vi "ziExample-QControl.vi"() -> ()   [LabVIEW 2009]
doc: "Control a Zurich instrument device via the LabOne Labview API. \nRequirements: Zurich Instruments HF2LI with HF2-MF and HF2-PID options.\nThis LabVIEW vi helps in configuring an HF2 to do Q-Control.\n\n© Zurich Instruments AG, www.zhinst.com"
uses:
  <instrlib>/Zurich Instruments LabOne/Public/Configure/ziSetValueDouble.vi
  <vilib>/Analysis/NI_AALPro.lvlib
  <vilib>/Utility/NIReport.llb/NI_report.lvclass
  <instrlib>/Zurich Instruments LabOne/Zurich Instruments LabOne.lvlib
panel:
  in  "restore settings":bool caption="Restore original settings"
  out "fmax":dbl=1000.0
  out "fmin":dbl=1000.0
  in  "Tab Control Sweep":enum32{"Sweeper", "Sweeper Settings", "Help"}(tab)
  in  "Drive (V)":dbl=0.01 format="%_3p"
  out "Resonance Frequency Q":dbl
  in  "Run Sweep":bool
  out "Sweep Progress":dbl(slide) max=21.0 scale=0.0..1.0
  out "Graph Phase":T1(graph)=[{"Output (F,X1,Y1,X2,Y2,...,Vo)"=[1841839.1959798995, 1841849.2462311557, 1841859.2964824121, 1841869.3467336684, 1841879.3969849246, 1841889.447236181, 1841899.4974874372, 1841909.5477386934, 1841919.5979899496, 1841929.648241206, 1841939.6984924623, 1841949.7487437185, 1841959.798994975, 1841969.8492462311, 1841979.8994974873, 1841989.9497487438, 1842000.0, 1842010.0502512562, 1842020.1005025127, 1842030.1507537689, 1842040.201005025, 1842050.2512562815, 1842060.3015075377, 1842070.351758794, 1842080.4020100501, 1842090.4522613066, 1842100.5025125628, 1842110.552763819, 1842120.6030150754, 1842130.6532663316, 1842140.7035175879, 1842150.7537688443, 1842160.8040201005, 1842170.8542713567, 1842180.9045226132, 1842190.9547738694, 1842201.0050251256, 1842211.055276382, 1842221.1055276382, 1842231.1557788944, 1842241.2060301506, 1842251.256281407, 1842261.3065326633, 1842271.3567839195, 1842281.407035176, 1842291.4572864322, 1842301.5075376884, 1842311.5577889448, 1842321.608040201, 1842331.6582914572, 1842341.7085427137, 1842351.7587939699, 1842361.809045226, 1842371.8592964825, 1842381.9095477387, 1842391.959798995, 1842402.0100502511, 1842412.0603015076, 1842422.1105527638, 1842432.16080402, 1842442.2110552764, 1842452.2613065327, 1842462.3115577889, 1842472.3618090453, 1842482.4120603015, 1842492.4623115577, 1842502.5125628142, 1842512.5628140704, 1842522.6130653266, 1842532.6633165828, 1842542.7135678392, 1842552.7638190954, 1842562.8140703517, 1842572.864321608, 1842582.9145728643, 1842592.9648241205, 1842603.015075377, 1842613.0653266332, 1842623.1155778894, 1842633.1658291458, 1842643.216080402, 1842653.2663316582, 1842663.3165829147, 1842673.3668341709, 1842683.417085427, 1842693.4673366833, 1842703.5175879397, 1842713.567839196, 1842723.6180904522, 1842733.6683417086, 1842743.7185929648, 1842753.768844221, 1842763.8190954775, 1842773.8693467337, 1842783.9195979899, 1842793.9698492463, 1842804.0201005025, 1842814.0703517587, 1842824.1206030152, 1842834.1708542714, 1842844.2211055276, 1842854.2713567838, 1842864.3216080402, 1842874.3718592965, 1842884.4221105527, 1842894.472361809, 1842904.5226130653, 1842914.5728643215, 1842924.623115578, 1842934.6733668342, 1842944.7236180904, 1842954.7738693468, 1842964.824120603, 1842974.8743718592, 1842984.9246231157, 1842994.974874372, 1843005.025125628, 1843015.0753768843, 1843025.1256281408, 1843035.175879397, 1843045.2261306532, 1843055.2763819096, 1843065.3266331658, 1843075.376884422, 1843085.4271356785, 1843095.4773869347, 1843105.527638191, 1843115.5778894473, 1843125.6281407035, 1843135.6783919598, 1843145.7286432162, 1843155.7788944724, 1843165.8291457286, 1843175.8793969848, 1843185.9296482413, 1843195.9798994975, 1843206.0301507537, 1843216.0804020101, 1843226.1306532663, 1843236.1809045225, 1843246.231155779, 1843256.2814070352, 1843266.3316582914, 1843276.3819095478, 1843286.432160804, 1843296.4824120603, 1843306.5326633165, 1843316.582914573, 1843326.6331658291, 1843336.6834170853, 1843346.7336683418, 1843356.783919598, 1843366.8341708542, 1843376.8844221106, 1843386.9346733668, 1843396.984924623, 1843407.0351758795, 1843417.0854271357, 1843427.135678392, 1843437.1859296483, 1843447.2361809046, 1843457.2864321608, 1843467.336683417, 1843477.3869346734, 1843487.4371859296, 1843497.4874371858, 1843507.5376884423, 1843517.5879396985, 1843527.6381909547, 1843537.6884422111, 1843547.7386934673, 1843557.7889447236, 1843567.83919598, 1843577.8894472362, 1843587.9396984924, 1843597.9899497489, 1843608.040201005, 1843618.0904522613, 1843628.1407035175, 1843638.190954774, 1843648.2412060301, 1843658.2914572863, 1843668.3417085428, 1843678.391959799, 1843688.4422110552, 1843698.4924623116, 1843708.5427135678, 1843718.592964824, 1843728.6432160805, 1843738.6934673367, 1843748.743718593, 1843758.7939698494, 1843768.8442211056, 1843778.8944723618, 1843788.944723618, 1843798.9949748744, 1843809.0452261306, 1843819.0954773868, 1843829.1457286433, 1843839.1959798995], "dX/dt"=[-6.94293659208085, -7.039263365714603, -7.015747865746605, -7.022831577183382, -7.070140649231355, -7.097687461922305, -7.105617775743133, -7.187018771027357, -7.215555605807255, -7.209120372797453, -7.222963353111247, -7.2482145424437725, -7.336471988299522, -7.392871009974112, -7.404378015656745, -7.392520359287413, -7.520355608686046, -7.519542598388936, -7.550628880706965, -7.581504623203495, -7.613602056591421, -7.5885724211422065, -7.700014320037284, -7.728140979121345, -7.810709171761543, -7.784263466588973, -7.881518062030821, -7.903674328964446, -7.971719351332499, -8.017529667992314, -8.058121436672986, -8.165785698106287, -8.19016022550502, -8.212700433959935, -8.32675261509468, -8.371215456694097, -8.455244319826404, -8.452589972505562, -8.593897328803308, -8.603598584374405, -8.66788383890823, -8.728838589412112, -8.92008246055265, -8.96248928060953, -9.014325061381626, -9.12099819745259, -9.192260387685824, -9.25577287991073, -9.393754573052911, -9.510460418962696, -9.588798588744128, -9.671919305255168, -9.807909390069907, -9.872318951901494, -10.029523543826793, -10.111178612582068, -10.282365199143047, -10.41392827403316, -10.600908552099941, -10.721664299953895, -10.861537419641733, -11.05386683133099, -11.226967260541015, -11.399833261360014, -11.614266576451872, -11.822489241822097, -12.037591738878548, -12.284275795570396, -12.537696676929697, -12.808591866080967, -13.10897592112657, -13.414554360121997, -13.74678013981217, -14.102456694459267, -14.476936500710565, -14.894674114827959, -15.339877668460199, -15.812096714688613, -16.374409982820275, -16.9513079644051, -17.5854888581396, -18.28427561683263, -19.054069906143813, -19.928879874410452, -20.90995289279427, -21.975478569369823, -23.22079284159497, -24.61324931082536, -26.23607602255107, -28.12290317293296, -30.316540859101774, -32.93351414204068, -36.0685114581311, -39.86225308894581, -44.52062048412513, -50.265070638918324, -57.397192144852305, -66.16528396414377, -76.63221848917898, -88.4706687072364, -100.82403856696656, -112.6132379050097, -122.9993546962758, -131.68277440223207, -138.73027439508525, -144.42272136521782, -149.00962859772702, -152.74574201067415, -155.83478009073983, -158.4057569715815, -160.55712878950192, -162.41389955531858, -163.98916270213934, -165.35435338829546, -166.5502332885727, -167.6188034018421, -168.54149862098475, -169.38780172777604, -170.13679818450444, -170.78748418559624, -171.41172295788104, -171.99098890699028, -172.50066268325997, -172.9556325234782, -173.4008952713357, -173.82760697801268, -174.17343776744914, -174.55598606411053, -174.82677313412782, -175.20114654856826, -175.44438260372488, -175.74183048219098, -176.00347473058068, -176.23123546164112, -176.43388652935894, -176.62506543519825, -176.8656495868036, -177.000286426292, -177.2712077683475, -177.36028159834026, -177.53319063513797, -177.67555828450963, -177.84294696805748, -178.0118748631806, -178.16232009535963, -178.27551219372313, -178.39423075255817, -178.4903282214428, -178.5715733424731, -178.73836280736876, -178.82943056728186, -178.9850843467714, -179.04192894715334, -179.08270482893664, -179.19287748311572, -179.28322843883868, -179.34165759880761, -179.50709018669053, -179.4954309299658, -179.64736857972363, -179.60928252514617, -179.78420449956272, -179.8065606796536, -179.84218357544378, -179.90164268987297, -179.9062773498495, -180.0402030141334, -180.21011520251875, -180.02003421747088, -180.17501517626974, -180.197905755971, -180.35296807746022, -180.37609298337136, -180.54331181359302, -180.49811587577673, -180.50365280444166, -180.6359768081795, -180.47976323601006, -180.5713600449198, -180.67329316815656, -180.6154046528325, -180.75094639042254, -180.5940820677559, -180.83667931766678, -180.72000977161738, -180.90668274161465, -180.88415063790313, -180.91032933351386, -180.93791455694205, -180.8862600292335, -180.9706632041318, -181.0058055371726, -181.12385131631882, -180.99226180353708, -181.17117500602515, -181.20440954183448, -181.1560016539221, -181.11269108982725, -181.29568987605847, -181.260867961045]}, {"Output (F,X1,Y1,X2,Y2,...,Vo)"=array[500 elements], "dX/dt"=array[500 elements]}] caption="Graph2"
  out "Graph Amplitude":T2(graph)=[{"Output (F,X1,Y1,X2,Y2,...,Vo)"=[1841839.1959798995, 1841849.2462311557, 1841859.2964824121, 1841869.3467336684, 1841879.3969849246, 1841889.447236181, 1841899.4974874372, 1841909.5477386934, 1841919.5979899496, 1841929.648241206, 1841939.6984924623, 1841949.7487437185, 1841959.798994975, 1841969.8492462311, 1841979.8994974873, 1841989.9497487438, 1842000.0, 1842010.0502512562, 1842020.1005025127, 1842030.1507537689, 1842040.201005025, 1842050.2512562815, 1842060.3015075377, 1842070.351758794, 1842080.4020100501, 1842090.4522613066, 1842100.5025125628, 1842110.552763819, 1842120.6030150754, 1842130.6532663316, 1842140.7035175879, 1842150.7537688443, 1842160.8040201005, 1842170.8542713567, 1842180.9045226132, 1842190.9547738694, 1842201.0050251256, 1842211.055276382, 1842221.1055276382, 1842231.1557788944, 1842241.2060301506, 1842251.256281407, 1842261.3065326633, 1842271.3567839195, 1842281.407035176, 1842291.4572864322, 1842301.5075376884, 1842311.5577889448, 1842321.608040201, 1842331.6582914572, 1842341.7085427137, 1842351.7587939699, 1842361.809045226, 1842371.8592964825, 1842381.9095477387, 1842391.959798995, 1842402.0100502511, 1842412.0603015076, 1842422.1105527638, 1842432.16080402, 1842442.2110552764, 1842452.2613065327, 1842462.3115577889, 1842472.3618090453, 1842482.4120603015, 1842492.4623115577, 1842502.5125628142, 1842512.5628140704, 1842522.6130653266, 1842532.6633165828, 1842542.7135678392, 1842552.7638190954, 1842562.8140703517, 1842572.864321608, 1842582.9145728643, 1842592.9648241205, 1842603.015075377, 1842613.0653266332, 1842623.1155778894, 1842633.1658291458, 1842643.216080402, 1842653.2663316582, 1842663.3165829147, 1842673.3668341709, 1842683.417085427, 1842693.4673366833, 1842703.5175879397, 1842713.567839196, 1842723.6180904522, 1842733.6683417086, 1842743.7185929648, 1842753.768844221, 1842763.8190954775, 1842773.8693467337, 1842783.9195979899, 1842793.9698492463, 1842804.0201005025, 1842814.0703517587, 1842824.1206030152, 1842834.1708542714, 1842844.2211055276, 1842854.2713567838, 1842864.3216080402, 1842874.3718592965, 1842884.4221105527, 1842894.472361809, 1842904.5226130653, 1842914.5728643215, 1842924.623115578, 1842934.6733668342, 1842944.7236180904, 1842954.7738693468, 1842964.824120603, 1842974.8743718592, 1842984.9246231157, 1842994.974874372, 1843005.025125628, 1843015.0753768843, 1843025.1256281408, 1843035.175879397, 1843045.2261306532, 1843055.2763819096, 1843065.3266331658, 1843075.376884422, 1843085.4271356785, 1843095.4773869347, 1843105.527638191, 1843115.5778894473, 1843125.6281407035, 1843135.6783919598, 1843145.7286432162, 1843155.7788944724, 1843165.8291457286, 1843175.8793969848, 1843185.9296482413, 1843195.9798994975, 1843206.0301507537, 1843216.0804020101, 1843226.1306532663, 1843236.1809045225, 1843246.231155779, 1843256.2814070352, 1843266.3316582914, 1843276.3819095478, 1843286.432160804, 1843296.4824120603, 1843306.5326633165, 1843316.582914573, 1843326.6331658291, 1843336.6834170853, 1843346.7336683418, 1843356.783919598, 1843366.8341708542, 1843376.8844221106, 1843386.9346733668, 1843396.984924623, 1843407.0351758795, 1843417.0854271357, 1843427.135678392, 1843437.1859296483, 1843447.2361809046, 1843457.2864321608, 1843467.336683417, 1843477.3869346734, 1843487.4371859296, 1843497.4874371858, 1843507.5376884423, 1843517.5879396985, 1843527.6381909547, 1843537.6884422111, 1843547.7386934673, 1843557.7889447236, 1843567.83919598, 1843577.8894472362, 1843587.9396984924, 1843597.9899497489, 1843608.040201005, 1843618.0904522613, 1843628.1407035175, 1843638.190954774, 1843648.2412060301, 1843658.2914572863, 1843668.3417085428, 1843678.391959799, 1843688.4422110552, 1843698.4924623116, 1843708.5427135678, 1843718.592964824, 1843728.6432160805, 1843738.6934673367, 1843748.743718593, 1843758.7939698494, 1843768.8442211056, 1843778.8944723618, 1843788.944723618, 1843798.9949748744, 1843809.0452261306, 1843819.0954773868, 1843829.1457286433, 1843839.1959798995], [-28.966250862681054, -28.908176655273337, -28.864467111398284, -28.808136126619875, -28.754602779877295, -28.681537195962324, -28.60547886691201, -28.542769551012277, -28.47986278834069, -28.413059310021236, -28.35033543586046, -28.29138537216195, -28.227086468764178, -28.15168084424244, -28.083132309459675, -28.006652538062877, -27.923391524657678, -27.862916544212467, -27.784208516740375, -27.70412391696607, -27.636354468592554, -27.55133643843743, -27.46146332129707, -27.389341692048106, -27.294868081757663, -27.219310281261595, -27.123230188479226, -27.03474855024407, -26.950586594813416, -26.85355121081612, -26.765683710166535, -26.675242143760556, -26.564063048008382, -26.474632733618588, -26.37565770196402, -26.280112494285053, -26.172991235949205, -26.072598624000236, -25.959534728054443, -25.860640493819343, -25.7465174301761, -25.631539306182212, -25.498858352667277, -25.39010824649092, -25.25774799718558, -25.142249321882026, -25.00555406360646, -24.887022970441244, -24.75211169976204, -24.617521743246748, -24.48274082231197, -24.3428232828688, -24.196009592241655, -24.047554642475653, -23.889297411413008, -23.739575356461376, -23.570294117173674, -23.41322125110465, -23.224954797726845, -23.058866498583328, -22.88382952274905, -22.69856576681898, -22.50867999213655, -22.31450162319383, -22.111370069423263, -21.90338344600061, -21.68504571797671, -21.461764169109074, -21.226543135169543, -20.99229287484784, -20.741801499413626, -20.479366183700762, -20.21176825406491, -19.937742640458776, -19.648956986305464, -19.3468251889951, -19.033496520395904, -18.701812675964042, -18.355682042916765, -17.99270040419432, -17.615604660651464, -17.21865908953786, -16.797539016940565, -16.356977304926286, -15.888200014085553, -15.391846986851675, -14.866834628179921, -14.309077261379437, -13.711689066706123, -13.074653632558586, -12.392712546398329, -11.663574717432795, -10.884371326060215, -10.054211061904741, -9.183959621011658, -8.284378130216394, -7.3946969716815065, -6.579866401883259, -5.946660172340811, -5.612275426625389, -5.660939792976745, -6.092597885403304, -6.819063594921346, -7.720596881253953, -8.692845639671399, -9.676601274917646, -10.63194093311314, -11.542743236475578, -12.406298891129273, -13.216035317601213, -13.98028024462563, -14.699677218013587, -15.379521411615144, -16.023339805333272, -16.632012788033276, -17.212135663274463, -17.763951487592156, -18.287404341430125, -18.79046016208909, -19.273915407845625, -19.736440474832023, -20.179725827914766, -20.608959575656495, -21.018134587427294, -21.422995318238737, -21.807627924716133, -22.17859768043806, -22.532821774822636, -22.88528270717979, -23.228299264102954, -23.55688511871147, -23.881717376684854, -24.19613894993444, -24.49895105674716, -24.802029226261308, -25.099837529936202, -25.392446478391577, -25.673862567600672, -25.947515476929528, -26.22420324643256, -26.473552872567087, -26.742550094460967, -27.00104527827544, -27.248345780939687, -27.491641603363373, -27.74480782051559, -27.98078562862448, -28.223226877341677, -28.4458543248418, -28.668372965623256, -28.91316733771661, -29.134686427564475, -29.34772484111448, -29.55621510607997, -29.784051895982245, -30.00136613401197, -30.219876575206612, -30.42218292074636, -30.618607334447535, -30.831568097485093, -31.031377814888664, -31.230073398030804, -31.42672173766795, -31.62404980158688, -31.819935098980814, -32.01368910890594, -32.20561075361435, -32.396695113595065, -32.58604024745495, -32.754436974363834, -32.96100063832588, -33.124166975360936, -33.323942883117475, -33.50090098141094, -33.683801355462585, -33.87460045378752, -34.03049976000201, -34.25189149349637, -34.40356326157614, -34.580744989166725, -34.75748170316221, -34.94748867729741, -35.11731073350964, -35.288783018518025, -35.44821022332193, -35.6213094778834, -35.8056140321162, -35.95929649243196, -36.124591783023774, -36.30593369611333, -36.503240497902596, -36.64816967067446, -36.79128348867193, -36.99164183710858, -37.143384953777364, -37.26823219562254, -37.49034966949507, -37.662154614518144, -37.81959794162762, -38.00695446481112]}, {"Output (F,X1,Y1,X2,Y2,...,Vo)"=array[500 elements], array[500 elements]}] caption="Graph1"
  out "Q Factor":dbl format="%_4f"
  out "Resonance Freq (Hz)":dbl
  out "Phase Shift (°)":dbl format="%#.2f"
  out "controlled":dbl format="%_4f"
  out "Gain Margin (dB)":dbl caption="native" format="%.2f"
  out "f/2Q (Hz)":dbl
  out "Characteristic Frequency Q":dbl
  in  "Output Demod":i32(ring)=6 items=["1", "2", "3", "4", "5", "6", "7", "8"]
  in  "Steps":dbl=100.0
  in  "BW (Hz)":dbl=500.0
  in  "AutoBW":bool caption="Auto"
  in  "Sweep Oscillator":i32(ring) caption="Oscillator" items=["1", "2", "3", "4", "5", "6"]
  in  "Show Derivative and Filter":bool caption="Show demodulator filter and phase derivative in graphs"
  in  "Tab Control QControl":T3(tab)
  in  "PID Drive Limit (V)":dbl=10.0 format="%.3g"
  in  "Center Frequency (Hz)":dbl=1000000.0 format="%#_8p"
  in  "Bandwidth (Hz)":dbl=1000.0 format="%#_4p"
  in  "Q Control En":bool caption="Enable"
  in  "HW Channel":i32(ring) caption="Signal Input and Output" items=["1", "2"]
  in  "Q Enhancement":dbl(slide) scale=0.1..100.0 scale format="%#_4g"
  in  "AutoCenter":bool caption="Auto Center"
  in  "Address":string="DEV"
  out "Selected Device":string
  in  "PIDs":i32(ring) items=["1 and 2", "3 and 4"]
  in  "Oscillator":i32(ring)=2 items=["1", "2", "3", "4", "5", "6"]
  in  "Feedback Phase (deg)":dbl(slide) scale=-180.0..180.0
  in  "Feedback Gain (V/Vrms)":dbl(slide) scale=0.01..100.0
  out "Stability Warning":bool
  in  "AutoPhase":bool caption="Auto"
  in  "Auto Gain":bool caption="Auto"
  out "ADC Over":bool
  in  "stop":bool
  # "Requires HF2LI or MFLI with MF and PID options."
  # "Beta user help:\n1) Connect the resonator to either Signal Output 1 and Signal Input 1 or to both #2.\n\n2) Find out the approximate resonator resonance frequency and enter it to the field \"Center Frequency\"\n\n3) Specify \"Bandwidth\" to be about 5x the width of the resonance peak (*).\n\n4) Start a sweep to find the native (natural) behavior of the resonator. The exact resonance frequency, Q-factor, characteristic frequency, phase at resonance and gain margin will be extracted. These values are crucial for a proper Q enhancement. (**)\n\n5) Set the \"Q Enhancement\" slider to the desired value (2 increases Q by a factor of two) and enable Q control.\n\n6) Start another sweep and compare the transfer functions.\n\n* Keep in mind that the resonance may not shift more than the Q-control bandwidth. Bandwidth should not be set to a higher value than 10kHz as the PID controllers can update the drive with about 100kHz.\n** The time constant setting for the sweeper should suit the characteristic frequency of the cantilever."
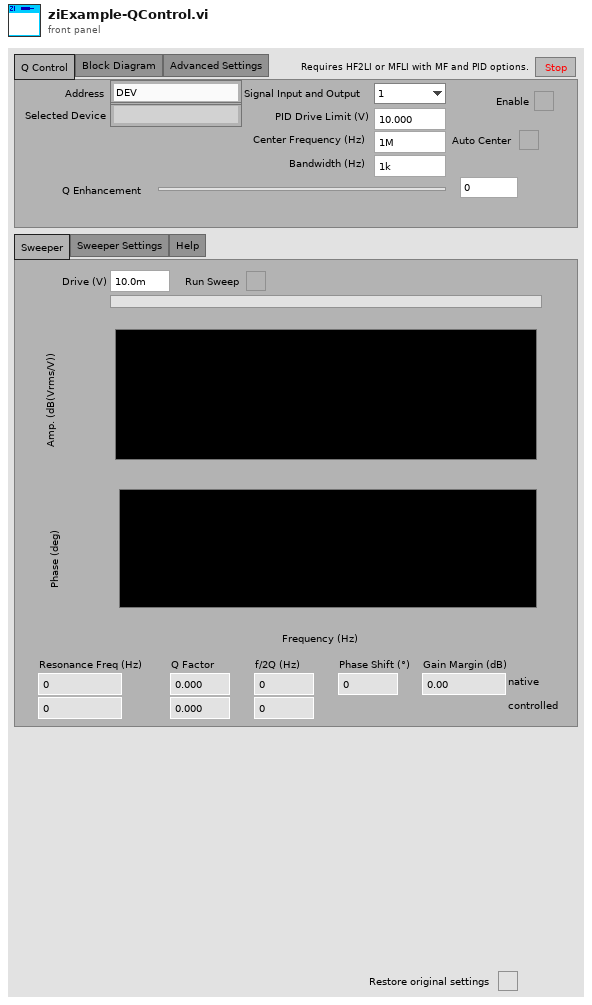
[diagram p1: front panel]
types:
  T1 = cluster{"Output (F,X1,Y1,X2,Y2,...,Vo)":dbl[], "dX/dt":dbl[]}[]
  T2 = cluster{"Output (F,X1,Y1,X2,Y2,...,Vo)":dbl[], dbl[]}[]
  T3 = enum32{"Q Control", "Block Diagram", "Advanced Settings"}
  T4 = enum32{"Page Enabled", "Page Disabled", "Page Disabled & Grayed"}
  T5 = enum8{"Enabled", "Disabled", "Disabled and Grayed Out"}
  T6 = typedef "Zurich Instruments LabOne.lvlib/ziTypeHandle.ctl" = cluster{"handleValid":bool, "Conn":u64, "Path Prefix":string, "Handle":u64, "Connected":bool, "Clockbase(s)":dbl}
  T7 = enum16{"Standard Report", "HTML", "Word", "Excel"}
  T8 = cluster{"Output (F,X1,Y1,X2,Y2,...,Vo)":dbl[], dbl[]}
  T9 = cluster{"Output (F,X1,Y1,X2,Y2,...,Vo)":dbl[], "Unwrapped Phase":dbl[]}
  T10 = enum32{"invalid app kind", "Development System", "Run Time System", "Student Edition", "Embedded LabVIEW", "Evaluation", "Custom"}
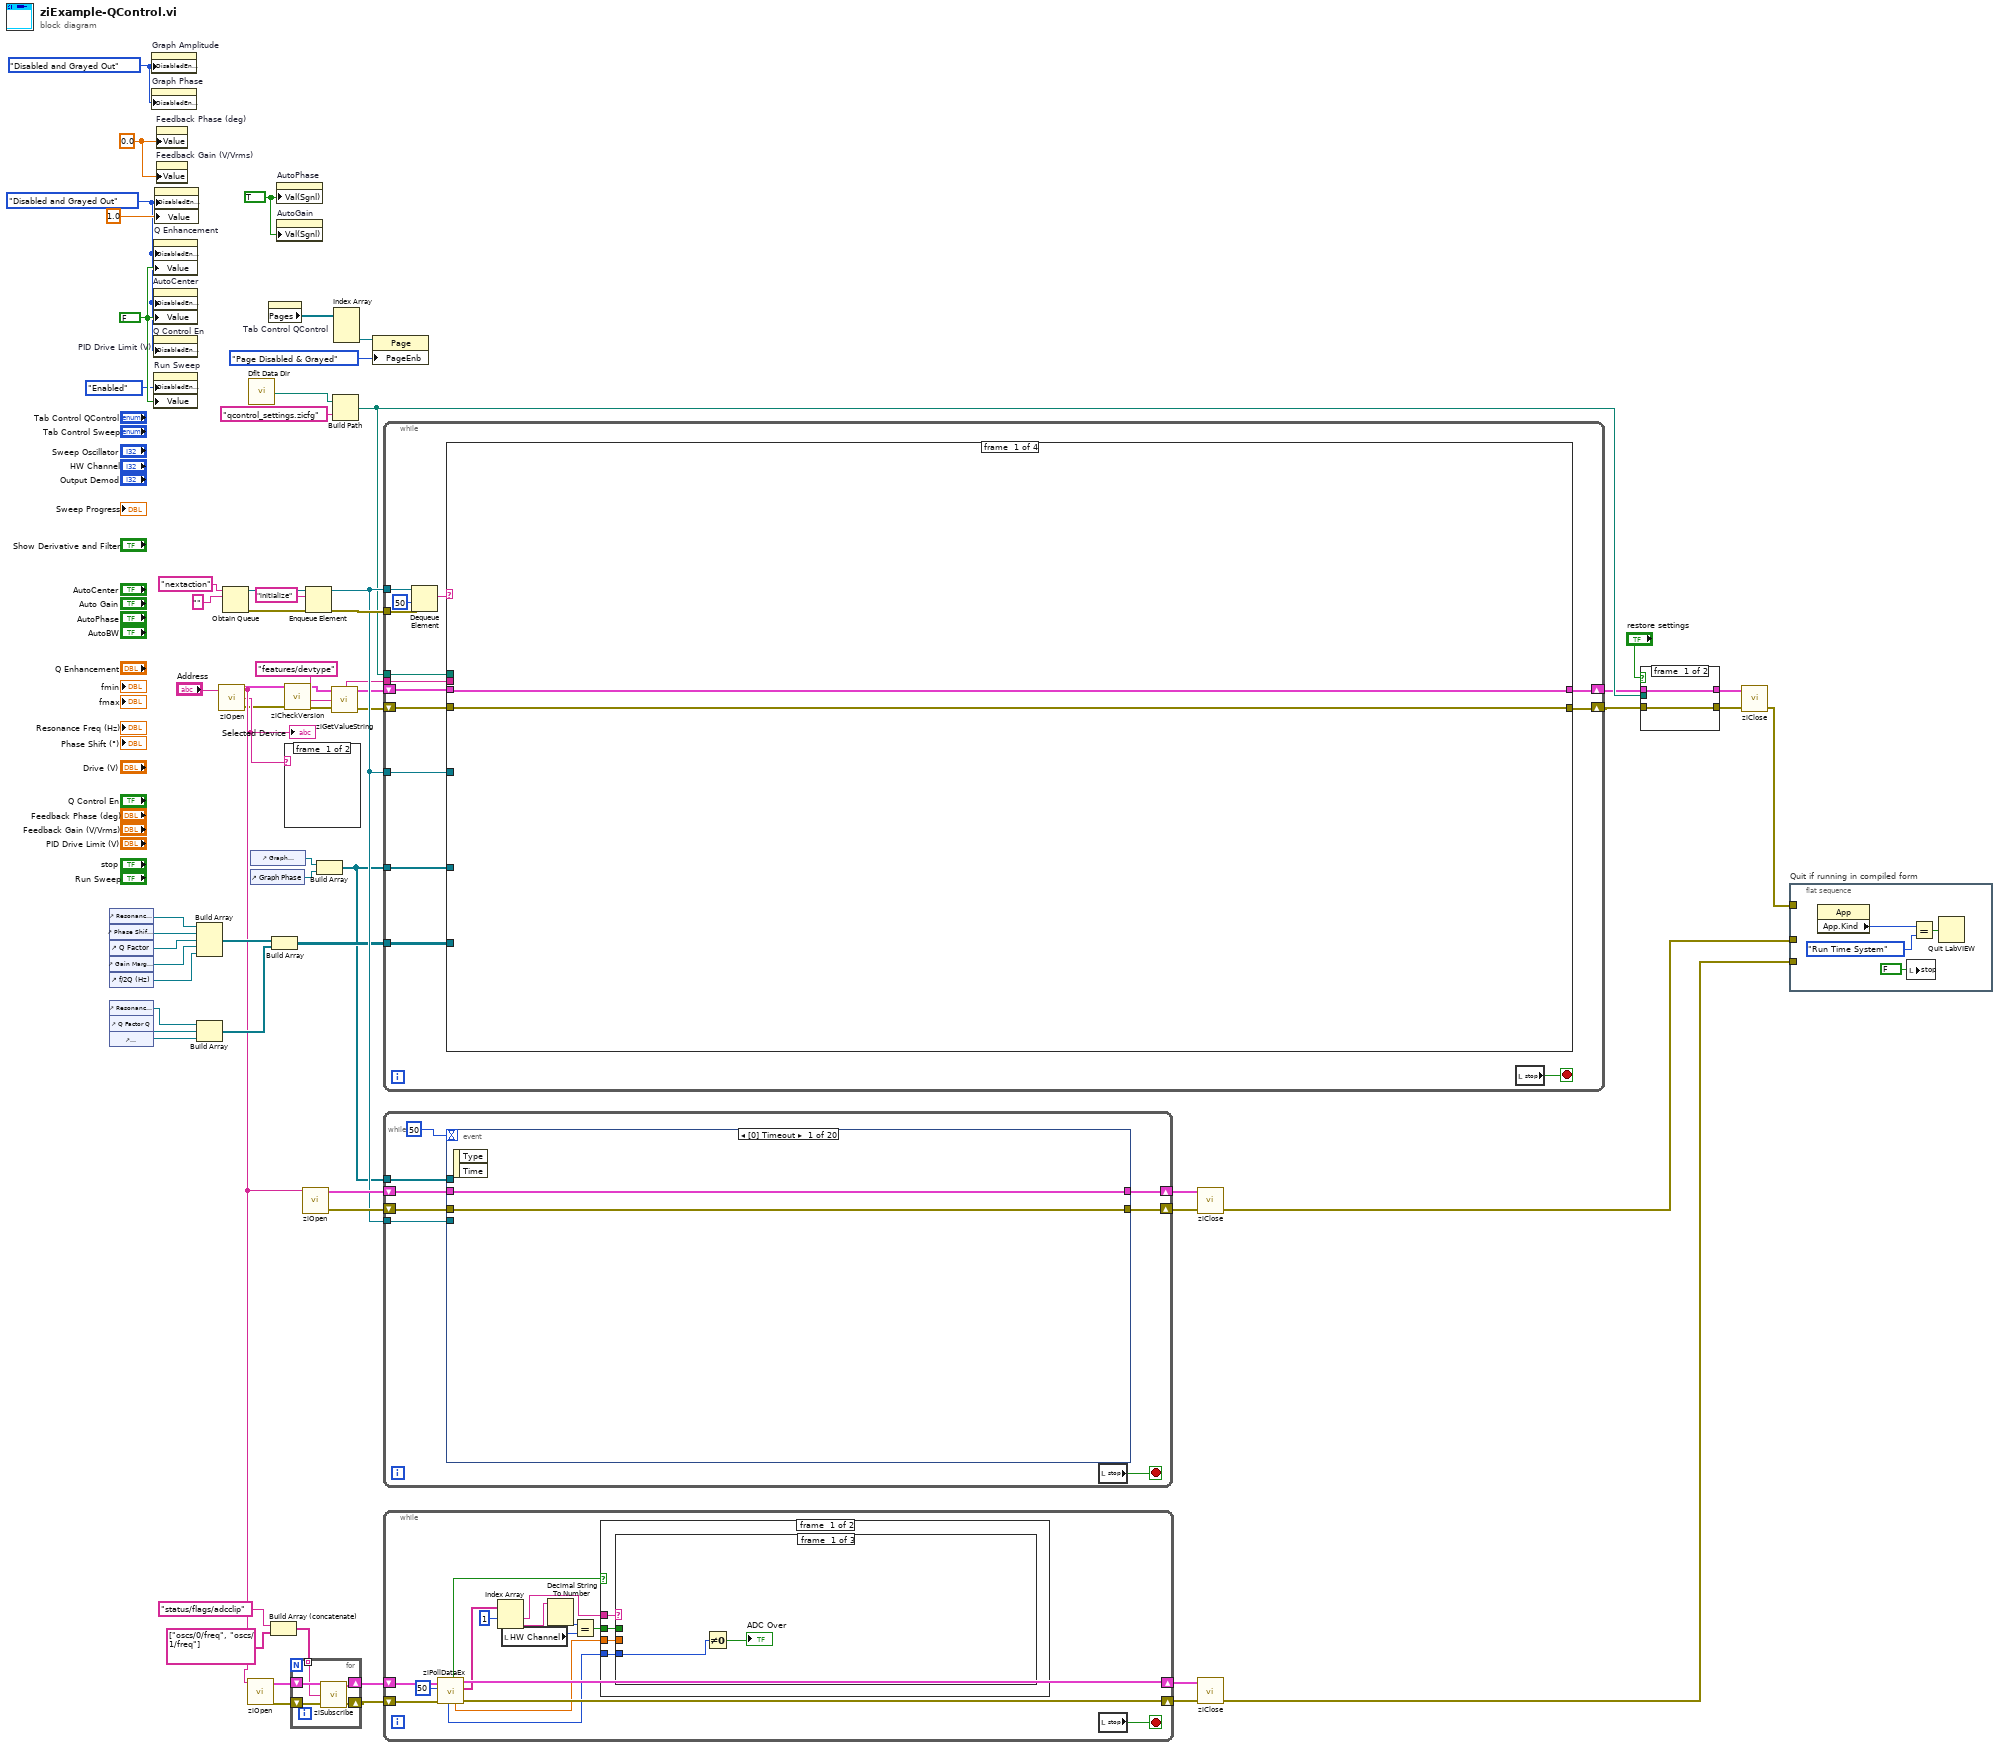
[diagram p0: block diagram]
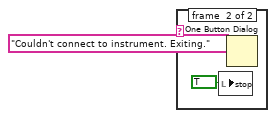
[diagram p2: hidden frame]
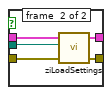
[diagram p3: hidden frame]
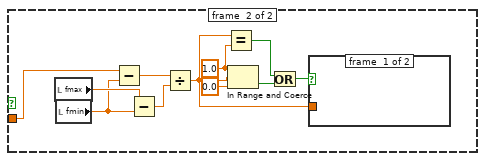
[diagram p6: hidden frame]
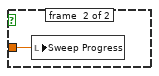
[diagram p7: hidden frame]
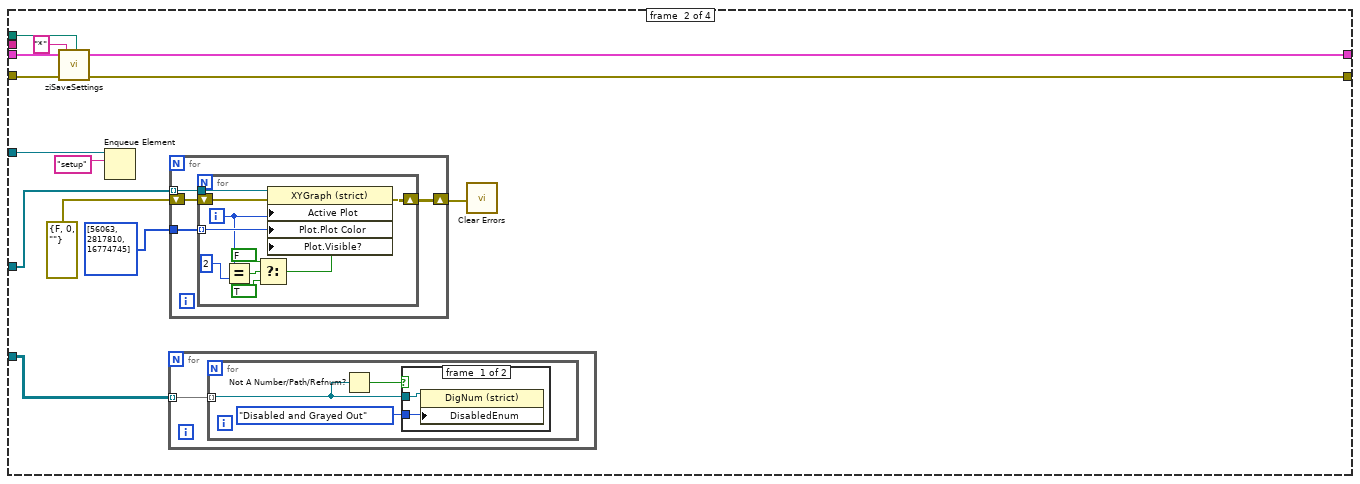
[diagram p9: hidden frame]
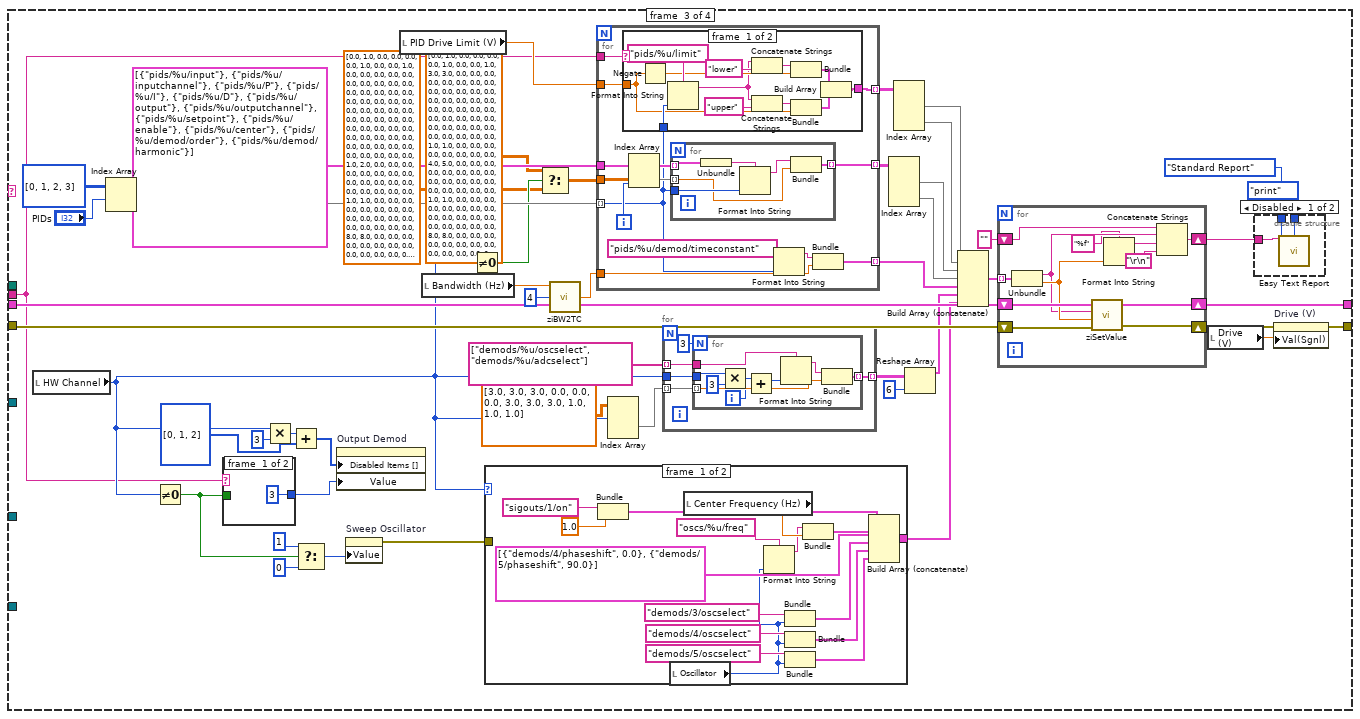
[diagram p11: hidden frame]
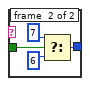
[diagram p12: hidden frame]
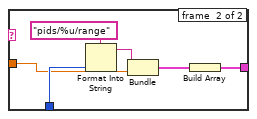
[diagram p14: hidden frame]
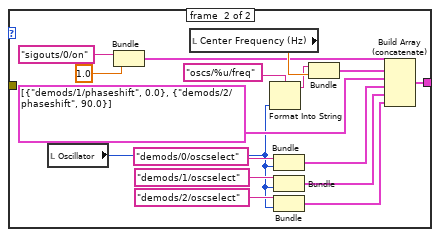
[diagram p15: hidden frame]
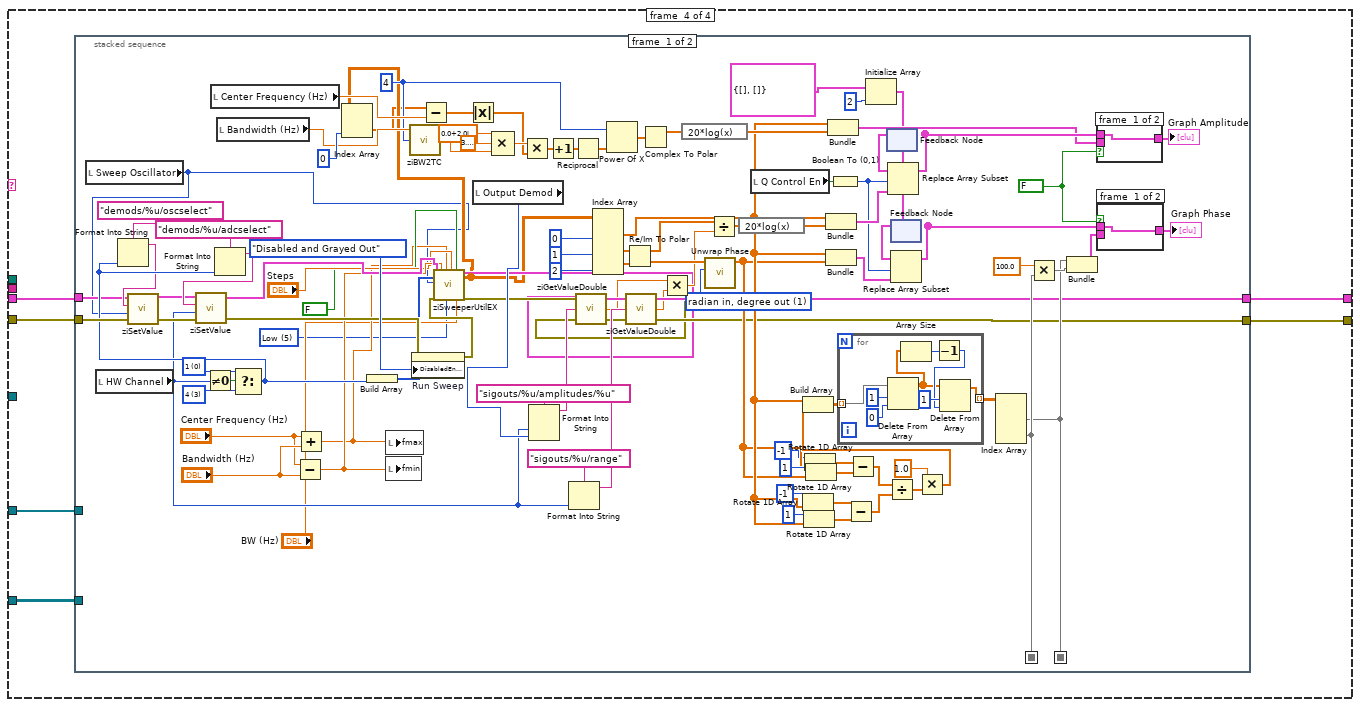
[diagram p16: hidden frame]
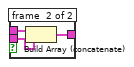
[diagram p17: hidden frame]
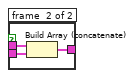
[diagram p18: hidden frame]
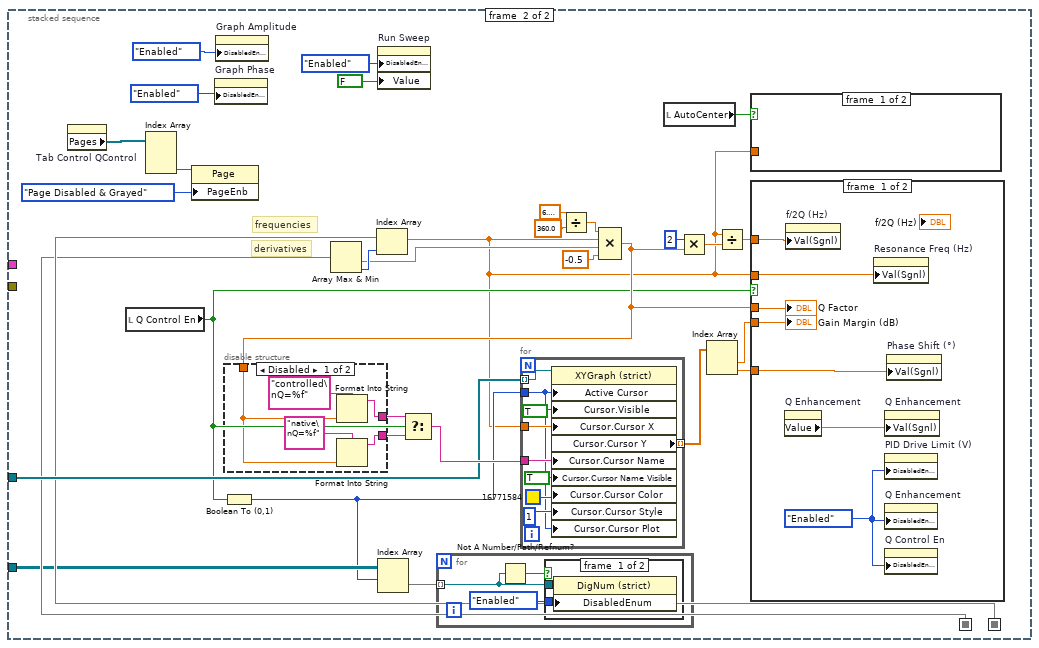
[diagram p19: hidden frame]
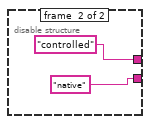
[diagram p20: hidden frame]
diagram:
  w6 = T5."Disabled and Grayed Out" ("Disabled")
  w17 = 0.0 ("Feedback Phase (deg)")
  w18 = TRUE ("AutoPhase")
  w5 = T5."Disabled and Grayed Out" ("Disabled")
  w20 = FALSE ("Q Control")
  n1 = control-ref of="Resonance Freq (Hz)"() -> (w50:refnum<vi>)
  n2 = control-ref of="Phase Shift (°)"() -> (w49:refnum<vi>)
  n3 = control-ref of="Q Factor"() -> (w48:refnum<vi>)
  n4 = control-ref of="Gain Margin (dB)"() -> (w47:refnum<vi>)
  n5 = control-ref of="f/2Q (Hz)"() -> (w40:refnum<vi>)
  n6 = control-ref of="Resonance Frequency Q"() -> (w38:refnum<vi>)
  n7 = control-ref of="Q Factor Q"() -> (w46:refnum<vi>)
  n8 = control-ref of="Characteristic Frequency Q"() -> (w39:refnum<vi>)
  n9 = property on="Graph Amplitude" class="XYGraph (strict)"("DisabledEnum"=w6) -> ()  [unwired: 2 in, 2 out]
  n10 = property on="Graph Phase" class="XYGraph (strict)"("DisabledEnum"=w6) -> ()  [unwired: 2 in, 2 out]
  n11 = property on="AutoCenter" class="Bool (strict)"("DisabledEnum"=w5, "Value"=w20) -> ()  [unwired: 2 in, 2 out]
  n12 = property on="Q Control En" class="Bool (strict)"("DisabledEnum"=w5, "Value"=w20) -> ()  [unwired: 2 in, 2 out]
  n13 = property on="PID Drive Limit (V)" class="DigNum (strict)"("DisabledEnum"=w5) -> ()  [unwired: 2 in, 2 out]
  n14 = property on="Run Sweep" class="Bool (strict)"("DisabledEnum"=T5."Enabled" ("Disabled"), "Value"=w20) -> ()  [unwired: 2 in, 2 out]
  n15 = property on="Q Enhancement" class="Slide (strict)"("DisabledEnum"=w5, "Value"=1.0 ("Q Enhancement")) -> ()  [unwired: 2 in, 2 out]
  n16 = property on="Feedback Phase (deg)" class="Slide (strict)"("Value"=w17) -> ()  [unwired: 2 in, 2 out]
  n17 = property on="Feedback Gain (V/Vrms)" class="Slide (strict)"("Value"=w17) -> ()  [unwired: 2 in, 2 out]
  n18 = Build Array(w50, w49, w48, w47, w40) -> (w44:refnum<vi>[])
  n19 = Build Array(w38, w46, w39) -> (w45:refnum<vi>[])
  n20 = call <instrlib>:"ziOpen.vi"("Address"="Address") -> ("Error Out"=w1:errorcluster, "Selected Device"=w8:string, "HandleOut"=w2:T6)  [unwired: 3 in]
  "Selected Device" <- w8
  n21 = Obtain Queue(name (unnamed)="nextaction", element data type="") -> (queue out=w63:refnum<queue>, error out=w61:errorcluster)  [unwired: 3 in, 1 out]
  n22 = call <instrlib>:"ziOpen.vi"("Address"="Address") -> ("Error Out"=w51:errorcluster, "HandleOut"=w52:T6)  [unwired: 3 in, 1 out]
  n23 = call <vilib>:"Dflt Data Dir.vi"() -> ("App:Default Data Directory"=w37:path)
  n24 = control-ref of="Graph Phase"() -> (w41:refnum<vi>)
  n25 = control-ref of="Graph Amplitude"() -> (w42:refnum<vi>)
  n26 = property on="Tab Control QControl" class="TabCtl (strict)"() -> ("Pages"=w14:refnum<vi>[])  [unwired: 2 in, 2 out]
  n27 = Build Array (concatenate)("status/flags/adcclip" ("Path ()"), string[] ["oscs/0/freq", "oscs/1/freq"]) -> (w27:string[])
  n28 = Build Array(w44, w45) -> (w43:refnum<vi>[][])
  n29 = property on="AutoPhase" class="Bool (strict)"("Val(Sgnl)"=w18) -> ()  [unwired: 2 in, 2 out]
  n30 = property on="AutoGain" class="Bool (strict)"("Val(Sgnl)"=w18) -> ()  [unwired: 2 in, 2 out]
  n31 = call <instrlib>:"ziCheckVersion.vi"("Handle In"=w2, "Error In"=w1) -> ("Handle Out"=w4:T6, "Error Out"=w3:errorcluster)  [unwired: 11 in, 1 out]
  n32 = case shown="Default" w8 {
    frame #0 {
    }
    frame #1 {
      n33 = local write "stop"(TRUE ("stop")) -> ()
      n34 = One Button Dialog(message="Couldn't connect to instrument. Exiting.") -> ()  [unwired: 1 in, 1 out]
    }
  }
  n35 = for {
    tunnel: w27 -> [w68] mode=indexing
    shift-right: [w71] -> w25
    shift-left: w52 -> [w72]
    shift-right: [w70] -> w24
    shift-left: w51 -> [w69]
    n36 = call <instrlib>:"ziSubscribe.vi"("error in"=w69, "Path ()"=w68, "Handle In"=w72) -> ("error out"=w70:errorcluster, "Handle Out"=w71:T6)  [unwired: 1 in]
  }
  n37 = call <instrlib>:"ziOpen.vi"("Address"="Address") -> ("Error Out"=w57:errorcluster, "HandleOut"=w59:T6)  [unwired: 3 in, 1 out]
  n38 = Enqueue Element(queue=w63, element="initialize" ("notification"), error in (no error)=w61) -> (queue out=w55:refnum<queue>, error out=w60:errorcluster)  [unwired: 1 in, 1 out]
  n39 = Build Array(w42, w41) -> (w29:refnum<vi>[])
  n40 = call <instrlib>:"ziGetValueString.vi"("error in"=w3, "Path"="features/devtype", "Handle In"=w4) -> ("error out"=w10:errorcluster, "Value"=w9:string, "Handle Out"=w12:T6)
  n41 = Build Path(base path=w37, name or relative path="qcontrol_settings.zicfg") -> (appended path=w35:path)
  n42 = Index Array(array=w14) -> (element #3=w16:refnum<vi>)  [unwired: 3 in, 2 out]
  n43 = property class="Page"(reference=w16, "PageEnb"=T4."Page Disabled & Grayed" ("Page Enabled State")) -> ()  [unwired: 1 in, 2 out]
  n44 = while {
    tunnel: w55 -> [w85]
    tunnel: w60 -> [w83]
    tunnel: w55 -> [w81]
    tunnel: w43 -> [w80]
    shift-right: [w76] -> w34
    shift-left: w12 -> [w79]
    shift-right: [w77] -> w33
    shift-left: w10 -> [w78]
    tunnel: w29 -> [w75]
    tunnel: w35 -> [w74]
    tunnel: w9 -> [w73]
    stop <- w86 stop-if-true
    n45 = Dequeue Element(queue=w85, timeout in ms (-1)=50, error in (no error)=w83) -> (element=w84:string)  [unwired: 3 out]
    n46 = case shown="\"setup\"" w84 {
      tunnel: w81 -> [_ w100 _ _]
      tunnel: w80 -> [_ w99 _ w278]
      tunnel: w79 -> [w88 w93 w163 w277]
      tunnel: w78 -> [w87 w94 w162 w276]
      tunnel: [w87 w94 w142 w275] -> w77
      tunnel: [w88 w92 w161 w274] -> w76
      tunnel: w75 -> [_ w95 _ w273]
      tunnel: w74 -> [_ w90 _ _]
      tunnel: w73 -> [_ _ w123 _]
      frame #0 {
      }
      frame #1 {
        n47 = call <instrlib>:"ziSaveSettings.vi"("Path (\"\")"="*" ("Path"), "file path (dialog if empty)"=w90, "Handle In"=w93) -> ("Handle Out"=w92:T6)  [unwired: 1 in, 2 out]
        n48 = Enqueue Element(queue=w100, element="setup" ("notification")) -> ()  [unwired: 2 in, 3 out]
        n49 = for {
          tunnel: w99 -> [w115] mode=indexing
          n50 = for {
            tunnel: w115 -> [w116] mode=indexing
            n51 = Not A Number/Path/Refnum?(number/path/refnum=w116) -> (NaN/Path/Refnum?=w117:bool)
            n52 = case shown="True" w117 {
              tunnel: T5."Disabled and Grayed Out" ("Disabled") -> [w120 _]
              tunnel: w116 -> [w119 _]
              frame #0 {
                n53 = property class="DigNum (strict)"(reference=w119, "DisabledEnum"=w120) -> ()  [unwired: 1 in, 2 out]
              }
              frame #1 {
              }
            }
          }
        }
        n54 = for {
          tunnel: w95 -> [w104] mode=indexing
          tunnel: u32[] [56063, 2817810, 16774745] -> [w103]
          shift-right: [w101] -> w96
          shift-left: errorcluster {"status"=FALSE, "code"=0, "source"=""} ("error in (no error)") -> [w102]
          n55 = for {
            tunnel: w104 -> [w114]
            tunnel: w103 -> [w113] mode=indexing
            shift-right: [w111] -> w101
            shift-left: w102 -> [w112]
            i -> [w110]
            n56 = Equal?(x=w110, y=2) -> (x = y?=w108:bool)
            n57 = Select(t=FALSE ("Plot.Visible"), s=w108, f=TRUE ("Plot.Visible")) -> (s? t:f=w107:bool)
            n58 = property class="XYGraph (strict)"(reference=w114, error in=w112, "Active Plot"=w110, "Plot.Plot Color"=w113, "Plot.Visible?"=w107) -> (error out=w111:errorcluster)  [unwired: 1 out]
          }
        }
        n59 = call <vilib>:"Clear Errors.vi"("error in (no error)"=w96) -> ()  [unwired: 6 in, 1 out]
      }
      frame #2 {
        n60 = local read "HW Channel"() -> (w127:i32)
        n61 = Index Array(array=i32[][] [[0, 1], [2, 3]], index (row)="PIDs") -> (element=w165:i32[])  [unwired: 1 in]
        n62 = Not Equal To 0?(x=w127) -> (x != 0?=w130:bool)
        n63 = case shown="\"MFLI\", Default" w123 {
          tunnel: [3 w172] -> w134
          tunnel: w130 -> [_ w171]
          frame #0 {
          }
          frame #1 {
            n64 = Select(t=7, s=w171, f=6) -> (s? t:f=w172:i32)
          }
        }
        n65 = Multiply(x=w127, y=3) -> (x*y=w126:i32)
        n66 = Add(x=w126, y=i32[] [0, 1, 2] ("Disabled Items []")) -> (x+y=w128:i32[])
        n67 = Select(t=1, s=w130, f=0) -> (s? t:f=w131:i32)
        n68 = property on="Output Demod" class="Ring (strict)"("Disabled Items []"=w128, "Value"=w134) -> ()  [unwired: 2 in, 2 out]
        n69 = property on="Sweep Oscillator" class="Ring (strict)"("Value"=w131) -> (error out=w149:errorcluster)  [unwired: 2 in, 1 out]
        n70 = local read "PID Drive Limit (V)"() -> (w124:dbl)
        n71 = local read "Bandwidth (Hz)"() -> (w169:dbl)
        n72 = Not Equal To 0?(x=w127) -> (x != 0?=w152:bool)
        n73 = case shown="1" w127 {
          tunnel: [w253 w267] -> w141
          tunnel: w149 -> [_ _]
          frame #0 {
            n74 = Bundle("sigouts/1/on", "TC (s)"=1.0) -> (w243:cluster{string, "TC (s)":dbl})  [unwired: 1 in]
            n75 = local read "Oscillator"() -> (w241:i32)
            n76 = local read "Center Frequency (Hz)"() -> (w249:dbl)
            n77 = Format Into String(format string="oscs/%u/freq", w241) -> (resulting string=w247:string)  [unwired: 2 in, 1 out]
            n78 = Bundle("demods/3/oscselect", "Oscillator"=w241) -> (w252:cluster{string, "Oscillator":i32})  [unwired: 1 in]
            n79 = Bundle("demods/4/oscselect", "Oscillator"=w241) -> (w251:cluster{string, "Oscillator":i32})  [unwired: 1 in]
            n80 = Bundle("demods/5/oscselect", "Oscillator"=w241) -> (w250:cluster{string, "Oscillator":i32})  [unwired: 1 in]
            n81 = Bundle(w247, "Center Frequency (Hz)"=w249) -> (w246:cluster{string, "Center Frequency (Hz)":dbl})  [unwired: 1 in]
            n82 = Build Array (concatenate)(w243, w246, cluster{string, dbl}[] [{"demods/4/phaseshift", 0.0}, {"demods/5/phaseshift", 90.0}], w252, w251, w250) -> (w253:cluster{string, "Center Frequency (Hz)":dbl}[])
          }
          frame #1 {
            n83 = local read "Oscillator"() -> (w257:i32)
            n84 = Bundle("sigouts/0/on", "TC (s)"=1.0) -> (w259:cluster{string, "TC (s)":dbl})  [unwired: 1 in]
            n85 = local read "Center Frequency (Hz)"() -> (w271:dbl)
            n86 = Format Into String(format string="oscs/%u/freq", w257) -> (resulting string=w262:string)  [unwired: 2 in, 1 out]
            n87 = Bundle("demods/0/oscselect", "Oscillator"=w257) -> (w266:cluster{string, "Oscillator":i32})  [unwired: 1 in]
            n88 = Bundle("demods/1/oscselect", "Oscillator"=w257) -> (w265:cluster{string, "Oscillator":i32})  [unwired: 1 in]
            n89 = Bundle("demods/2/oscselect", "Oscillator"=w257) -> (w264:cluster{string, "Oscillator":i32})  [unwired: 1 in]
            n90 = Bundle(w262, "Center Frequency (Hz)"=w271) -> (w272:cluster{string, "Center Frequency (Hz)":dbl})  [unwired: 1 in]
            n91 = Build Array (concatenate)(w259, w272, cluster{string, dbl}[] [{"demods/1/phaseshift", 0.0}, {"demods/2/phaseshift", 90.0}], w266, w265, w264) -> (w267:cluster{string, "Center Frequency (Hz)":dbl}[])
          }
        }
        n92 = Select(t=dbl[][] [[0.0, 1.0, 0.0, 0.0, 0.0, 0.0, 1.0, 0.0, 0.0, 1.0], [3.0, 3.0, 0.0, 0.0, 0.0, 0.0, 0.0, 0.0, 0.0, 0.0], [0.0, 0.0, 0.0, 0.0, 0.0, 0.0, 0.0, 0.0, 0.0, 0.0], [0.0, 0.0, 0.0, 0.0, 0.0, 0.0, 0.0, 0.0, 0.0, 0.0], [0.0, 0.0, 0.0, 0.0, 0.0, 0.0, 0.0, 0.0, 0.0, 0.0], [1.0, 1.0, 0.0, 0.0, 0.0, 0.0, 0.0, 0.0, 0.0, 0.0], [4.0, 5.0, 0.0, 0.0, 0.0, 0.0, 0.0, 0.0, 0.0, 0.0], [0.0, 0.0, 0.0, 0.0, 0.0, 0.0, 0.0, 0.0, 0.0, 0.0], [1.0, 1.0, 0.0, 0.0, 0.0, 0.0, 0.0, 0.0, 0.0, 0.0], [0.0, 0.0, 0.0, 0.0, 0.0, 0.0, 0.0, 0.0, 0.0, 0.0], [8.0, 8.0, 0.0, 0.0, 0.0, 0.0, 0.0, 0.0, 0.0, 0.0], [0.0, 0.0, 0.0, 0.0, 0.0, 0.0, 0.0, 0.0, 0.0, 0.0]], s=w152, f=dbl[][] [[0.0, 1.0, 0.0, 0.0, 0.0, 0.0, 1.0, 0.0, 0.0, 1.0], [0.0, 0.0, 0.0, 0.0, 0.0, 0.0, 0.0, 0.0, 0.0, 0.0], [0.0, 0.0, 0.0, 0.0, 0.0, 0.0, 0.0, 0.0, 0.0, 0.0], [0.0, 0.0, 0.0, 0.0, 0.0, 0.0, 0.0, 0.0, 0.0, 0.0], [0.0, 0.0, 0.0, 0.0, 0.0, 0.0, 0.0, 0.0, 0.0, 0.0], [0.0, 0.0, 0.0, 0.0, 0.0, 0.0, 0.0, 0.0, 0.0, 0.0], [1.0, 2.0, 0.0, 0.0, 0.0, 0.0, 0.0, 0.0, 0.0, 0.0], [0.0, 0.0, 0.0, 0.0, 0.0, 0.0, 0.0, 0.0, 0.0, 0.0], [1.0, 1.0, 0.0, 0.0, 0.0, 0.0, 0.0, 0.0, 0.0, 0.0], [0.0, 0.0, 0.0, 0.0, 0.0, 0.0, 0.0, 0.0, 0.0, 0.0], [8.0, 8.0, 0.0, 0.0, 0.0, 0.0, 0.0, 0.0, 0.0, 0.0], [0.0, 0.0, 0.0, 0.0, 0.0, 0.0, 0.0, 0.0, 0.0, 0.0]]) -> (s? t:f=w151:dbl[][])
        n93 = call <instrlib>:"ziBW2TC.vi"("Order (1)"=4 ("Order (#)"), "BW (Hz)"=w169) -> ("TC (s)"=w146:dbl)  [unwired: 1 in]
        n94 = for {
          tunnel: w165 -> [w207] mode=indexing
          tunnel: cluster{string}[] [{"pids/%u/input"}, {"pids/%u/inputchannel"}, {"pids/%u/P"}, {"pids/%u/I"}, {"pids/%u/D"}, {"pids/%u/output"}, {"pids/%u/outputchannel"}, {"pids/%u/setpoint"}, {"pids/%u/enable"}, {"pids/%u/center"}, {"pids/%u/demod/order"}, {"pids/%u/demod/harmonic"}] -> [w216]
          tunnel: [w215] -> w159 mode=indexing
          tunnel: w151 -> [w214]
          tunnel: [w211] -> w150 mode=indexing
          tunnel: w146 -> [w210]
          tunnel: [w206] -> w145 mode=indexing
          tunnel: w123 -> [w205]
          tunnel: w124 -> [w204]
          i -> [w212]
          n95 = case shown="\"HF2LI\"" w205 {
            tunnel: [w218 w230] -> w211
            tunnel: w207 -> [w228 w233]
            tunnel: w204 -> [w224 w232]
            frame #0 {
              n96 = Negate(x=w224) -> (-x=w225:dbl)
              n97 = Format Into String(format string="pids/%u/limit", w228) -> (resulting string=w222:string)  [unwired: 2 in, 1 out]
              n98 = Concatenate Strings(w222, "lower") -> (w217:string)
              n99 = Concatenate Strings(w222, "upper") -> (w221:string)
              n100 = Bundle(w217, w225) -> (w220:cluster{string, dbl})  [unwired: 1 in]
              n101 = Bundle(w221, "PID Drive Limit (V)"=w224) -> (w219:cluster{string, "PID Drive Limit (V)":dbl})  [unwired: 1 in]
              n102 = Build Array(w220, w219) -> (w218:cluster{string, "PID Drive Limit (V)":dbl}[])
            }
            frame #1 {
              n103 = Format Into String(format string="pids/%u/range", w233) -> (resulting string=w234:string)  [unwired: 2 in, 1 out]
              n104 = Bundle(w234, "PID Drive Limit (V)"=w232) -> (w231:cluster{string, "PID Drive Limit (V)":dbl})  [unwired: 1 in]
              n105 = Build Array(w231) -> (w230:cluster{string, "PID Drive Limit (V)":dbl}[])
            }
          }
          n106 = Index Array(array=w214, index (col)=w212) -> (element=w213:dbl[])  [unwired: 1 in]
          n107 = for {
            tunnel: w216 -> [w236] mode=indexing
            tunnel: w207 -> [w239]
            tunnel: [w238] -> w215 mode=indexing
            tunnel: w213 -> [w237] mode=indexing
            n108 = Unbundle(w236) -> (w235:string)
            n109 = Format Into String(format string=w235, w239) -> (resulting string=w240:string)  [unwired: 2 in, 1 out]
            n110 = Bundle(w240, w237) -> (w238:cluster{string, dbl})  [unwired: 1 in]
          }
          n111 = Format Into String(format string="pids/%u/demod/timeconstant", w207) -> (resulting string=w209:string)  [unwired: 2 in, 1 out]
          n112 = Bundle(w209, "TC (s)"=w210) -> (w206:cluster{string, "TC (s)":dbl})  [unwired: 1 in]
        }
        n113 = Index Array(array=dbl[][][] [[[3.0, 3.0, 3.0], [0.0, 0.0, 0.0]], [[3.0, 3.0, 3.0], [1.0, 1.0, 1.0]]], index (dim 0)=w127) -> (element=w139:dbl[][])  [unwired: 2 in]
        n114 = for {
          tunnel: string[] ["demods/%u/oscselect", "demods/%u/adcselect"] -> [w178] mode=indexing
          tunnel: w139 -> [w177] mode=indexing
          tunnel: w127 -> [w176]
          tunnel: [w175] -> w137 mode=indexing
          n115 = for {
            N: 3 -> [_]
            tunnel: w178 -> [w185]
            tunnel: [w188] -> w175 mode=indexing
            tunnel: w177 -> [w186] mode=indexing
            tunnel: w176 -> [w182]
            i -> [w181]
            n116 = Multiply(x=w182, y=3) -> (x*y=w183:i32)
            n117 = Add(x=w183, y=w181) -> (x+y=w180:i32)
            n118 = Format Into String(format string=w185, w180) -> (resulting string=w187:string)  [unwired: 2 in, 1 out]
            n119 = Bundle(w187, w186) -> (w188:cluster{string, dbl})  [unwired: 1 in]
          }
        }
        n120 = Index Array(array=w159) -> (element #1=w158:cluster{string, dbl}[], element #2=w157:cluster{string, dbl}[])  [unwired: 4 in]
        n121 = Index Array(array=w150) -> (element #1=w121:cluster{string, "PID Drive Limit (V)":dbl}[], element #2=w122:cluster{string, "PID Drive Limit (V)":dbl}[])  [unwired: 4 in]
        n122 = Reshape Array(w137, 6 ("dimension size")) -> (w136:cluster{string, dbl}[])
        n123 = Build Array (concatenate)(w121, w122, w158, w157, w145, w136, w141) -> (w160:cluster{string, "Center Frequency (Hz)":dbl}[])
        n124 = for {
          tunnel: w160 -> [w199] mode=indexing
          shift-right: [w202] -> w161
          shift-left: w163 -> [w203]
          shift-right: [w200] -> w143
          shift-left: w162 -> [w201]
          shift-right: [w195] -> w156
          shift-left: "" -> [w194]
          n125 = Unbundle(w199) -> (w196:string, "Center Frequency (Hz)"=w198:dbl)
          n126 = call-poly <instrlib>:"ziSetValue.vi"("Error In"=w201, "Value"=w198, "Path"=w196, "Handle In"=w203) -> ("Error Out"=w200:errorcluster, "Handle Out"=w202:T6)  [unwired: 1 in]
          n127 = Format Into String(format string="%f" ("initial string"), w198) -> (resulting string=w197:string)  [unwired: 2 in, 1 out]
          n128 = Concatenate Strings(w194, w196, w197, "\r\n") -> (w195:string)
        }
        n129 = local read "Drive (V)"() -> (w144:dbl)
        n130 = disable-structure shown="Disabled" {
          disable-tunnel: w156 -> [w191 _]
          disable-tunnel: enum16{"print", "save"}."print" ("print or save? (Word/Excel/HTML)") -> [w190 _]
          disable-tunnel: T7."Standard Report" ("report type") -> [w189 _]
          frame #0 {
            n131 = call <vilib>:"Easy Text Report.vi"("text to be printed"=w191, "print or save? (Word/Excel/HTML)"=w190, "report type"=w189) -> ()  [unwired: 12 in, 1 out]
          }
          frame #1 {
          }
        }
        n132 = property on="Drive (V)" class="DigNum (strict)"(error in=w143, "Val(Sgnl)"=w144) -> (error out=w142:errorcluster)  [unwired: 1 in, 1 out]
      }
      frame #3 {
        n133 = stacked-sequence {
          seq-local: [w318 _] -> [_ w412]
          seq-local: [w319 _] -> [_ w411]
          tunnel: w278 -> [_ w410]
          tunnel: w277 -> [w300 _]
          tunnel: w276 -> [w306 _]
          tunnel: [w315 _] -> w275
          tunnel: [w316 _] -> w274
          tunnel: w273 -> [_ w414]
          frame #0 {
            w279 = 5 items=["Low"=5, "Medium"=15, "High"=50] ("Precision (Low)")
            w321 = 3 items=["1", "2", "3", "4", "5", "6"] ("Sweep Oscillator")
            w339 = FALSE
            w322 = 0 items=["1", "2", "3", "4", "5", "6"] ("Sweep Oscillator")
            w327 = 4 ("Order (#)")
            w377 = 1 items=["radian in, radian out", "radian in, degree out", "degree in, degree out", "degree in, radian out"] ("phase unit")
            n134 = local read "Sweep Oscillator"() -> (w280:i32)
            n135 = local read "HW Channel"() -> (w297:i32)
            n136 = Not Equal To 0?(x=w297) -> (x != 0?=w320:bool)
            n137 = local read "Center Frequency (Hz)"() -> (w359:dbl)
            n138 = local read "Bandwidth (Hz)"() -> (w358:dbl)
            n139 = Select(t=w322, s=w320, f=w321) -> (s? t:f=w302:i32)
            n140 = Format Into String(format string="demods/%u/oscselect", w302) -> (resulting string=w301:string)  [unwired: 2 in, 1 out]
            n141 = call-poly <instrlib>:"ziSetValue.vi"("Error In"=w306, "Value"=w280, "Path"=w301, "Handle In"=w300) -> ("Error Out"=w305:errorcluster, "Handle Out"=w304:T6)  [unwired: 1 in]
            n142 = Format Into String(format string="demods/%u/adcselect", w302) -> (resulting string=w307:string)  [unwired: 2 in, 1 out]
            n143 = call-poly <instrlib>:"ziSetValue.vi"("Error In"=w305, "Value"=w297, "Path"=w307, "Handle In"=w304) -> ("Error Out"=w299:errorcluster, "Handle Out"=w289:T6)  [unwired: 1 in]
            n144 = Subtract(x="Center Frequency (Hz)", y="Bandwidth (Hz)") -> (x-y=w286:dbl)
            n145 = Add(x="Center Frequency (Hz)", y="Bandwidth (Hz)") -> (x+y=w283:dbl)
            n146 = Build Array(w302) -> (w282:i32[])
            n147 = local write "fmax"(w283) -> ()
            n148 = local write "fmin"(w286) -> ()
            n149 = call <instrlib>:"ziBW2TC.vi"("Order (1)"=w327, "BW (Hz)"=w358) -> ("TC (s)"=w325:dbl)  [unwired: 1 in]
            n150 = property on="Run Sweep" class="Bool (strict)"(error in=w299, "DisabledEnum"=T5."Disabled and Grayed Out" ("Disabled")) -> (error out=w290:errorcluster)  [unwired: 1 in, 1 out]
            n151 = call <instrlib>:"ziSweeperUtilEX.vi"("Handle In"=w289, "Input Demods (0)"=w282, "Oscillator (0)"=w280, "Error In"=w290, "Start (Hz)"=w286, "Stop (Hz)"=w283, "Precision (Low)"=w279, "Steps (#)"="Steps", "Log Sweep (true)"=FALSE, "Bandwith (-1=auto)"="BW (Hz)") -> ("Handle Out"=w291:T6, "Output (F,X1,Y1,X2,Y2,...,Vo)"=w288:dbl[][], "Error Out"=w292:errorcluster)  [unwired: 7 in]
            n152 = Index Array(array=w288, index (col)=0 ("disabled index (col)")) -> (element=w287:dbl[])  [unwired: 1 in]
            n153 = Subtract(x=w287, y=w359) -> (x-y=w326:dbl[])
            n154 = Absolute Value(x=w326) -> (abs(x)=w329:dbl[])
            n155 = local read "Output Demod"() -> (w298:i32)
            n156 = Compound Arithmetic op=MULTIPLY(cdb 0.0+2.0i ("r * e^(i*theta)"), 3.141592653589793, w325) -> (w333:cdb)
            n157 = Multiply(x=w333, y=w329) -> (x*y=w330:cdb[])
            n158 = Format Into String(format string="sigouts/%u/amplitudes/%u" ("Cursor.Cursor Name"), w297, w298) -> (resulting string=w294:string)  [unwired: 2 in, 1 out]
            n159 = Increment(x=w330) -> (x+1=w332:cdb[])
            n160 = Format Into String(format string="sigouts/%u/range" ("Cursor.Cursor Name"), w297) -> (resulting string=w314:string)  [unwired: 2 in, 1 out]
            n161 = Reciprocal(x=w332) -> (1/x=w331:cdb[])
            n162 = call <instrlib>:"ziGetValueDouble.vi"("error in"=w292, "Path"=w294, "Handle in"=w291) -> ("error out"=w296:errorcluster, "Value"=w293:dbl, "Handle out"=w295:T6)
            n163 = Index Array(array=w288, index (col) #1=0 ("disabled index (col)"), index (col) #2=1 ("index (col)"), index (col) #3=2 ("index (col)")) -> (element #1=w352:dbl[], element #2=w384:dbl[], element #3=w383:dbl[])  [unwired: 3 in]
            n164 = Power Of X(1:w331, 2:w327) -> (0:w328:cdb[])
            n165 = Re/Im To Polar(2:w383, 3:w384) -> (0:w378:dbl[], 1:w338:dbl[])
            n166 = call <instrlib>:"ziGetValueDouble.vi"("error in"=w296, "Path"=w314, "Handle in"=w295) -> ("error out"=w315:errorcluster, "Value"=w312:dbl, "Handle out"=w316:T6)
            n167 = Complex To Polar(r * e^(i*theta)=w328) -> (r=w374:dbl[])  [unwired: 1 out]
            n168 = Multiply(x=w293, y=w312) -> (x*y=w313:dbl)
            n169 = expression code="20*log(x)"(w374) -> (w375:dbl[])
            n170 = call <vilib>:"Unwrap Phase.vi"("phase unit"=w377, "Phase"=w378) -> ("Unwrapped Phase"=w349:dbl[])  [unwired: 8 in, 1 out]
            n171 = Divide(x=w338, y=w313) -> (x/y=w337:dbl[])
            n172 = expression code="20*log(x)"(w337) -> (w379:dbl[])
            n173 = local read "Q Control En"() -> (w311:bool)
            n174 = Rotate 1D Array(1:w352, 2:-1 ("n")) -> (0:w353:dbl[])
            n175 = Rotate 1D Array(1:w352, 2:1 ("n")) -> (0:w369:dbl[])
            n176 = Rotate 1D Array(1:w349, 2:-1 ("n")) -> (0:w350:dbl[])
            n177 = Rotate 1D Array(1:w349, 2:1 ("n")) -> (0:w370:dbl[])
            n178 = Bundle("Output (F,X1,Y1,X2,Y2,...,Vo)"=w352, w379) -> (w354:T8)  [unwired: 1 in]
            n179 = Bundle("Output (F,X1,Y1,X2,Y2,...,Vo)"=w352, "Unwrapped Phase"=w349) -> (w342:T9)  [unwired: 1 in]
            n180 = Bundle("Output (F,X1,Y1,X2,Y2,...,Vo)"=w352, w375) -> (w347:T8)  [unwired: 1 in]
            n181 = Boolean To (0,1)(Boolean=w311) -> (0, 1=w310:i16)
            n182 = Subtract(x=w353, y=w369) -> (x-y=w366:dbl[])
            n183 = Subtract(x=w350, y=w370) -> (x-y=w367:dbl[])
            n184 = Initialize Array(cluster{dbl[], dbl[]} {[], []}, 2 ("dimension size")) -> (w343:cluster{dbl[], dbl[]}[])
            n185 = feedback #1(w343) -> (w345:cluster{dbl[], dbl[]}[])
            n186 = Divide(x=w367, y=w366) -> (x/y=w365:dbl[])
            n187 = Replace Array Subset(array=w345, new element=w354, index=w310) -> (w362:cluster{dbl[], dbl[]}[])
            n188 = feedback #2(w343) -> (w344:cluster{dbl[], dbl[]}[])
            n189 = Replace Array Subset(array=w344, new element=w342, index=w310) -> (w341:cluster{dbl[], dbl[]}[])
            n190 = Multiply(x=1.0 ("Timeconstant (s)"), y=w365) -> (x*y=w357:dbl[])
            n191 = Build Array(w352, w357) -> (w356:dbl[][])
            n192 = for {
              tunnel: w356 -> [w398] mode=indexing
              tunnel: [w393] -> w355 mode=indexing
              n193 = Delete From Array(array=w398, length=1, index=0) -> (array with subset deleted=w394:dbl[])  [unwired: 1 out]
              n194 = Array Size(array=w394) -> (size(s)=w396:i32)
              n195 = Decrement(x=w396) -> (x-1=w395:i32)
              n196 = Delete From Array(array=w394, length=1, index=w395) -> (array with subset deleted=w393:dbl[])  [unwired: 1 out]
            }
            n197 = Index Array(array=w355) -> (element #1=w318:dbl[], element #2=w319:dbl[])  [unwired: 4 in]
            n198 = Multiply(x=100.0 ("Timeconstant (s)"), y=w319) -> (x*y=w363:dbl[])
            n199 = Bundle(w318, w363) -> (w373:cluster{dbl[], dbl[]})  [unwired: 1 in]
            n200 = case shown="True" w339 {
              tunnel: w362 -> [w385 w388]
              tunnel: w347 -> [_ w386]
              tunnel: [w385 w387] -> w346
              frame #0 {
              }
              frame #1 {
                n201 = Build Array (concatenate)(w388, w386) -> (w387:T2)
              }
            }
            "Graph Amplitude" <- w346
            n202 = case shown="False" w339 {
              tunnel: w373 -> [_ w392]
              tunnel: [w389 w391] -> w372
              tunnel: w341 -> [w389 w390]
              frame #0 {
              }
              frame #1 {
                n203 = Build Array (concatenate)(w390, w392) -> (w391:cluster{dbl[], dbl[]}[])
              }
            }
            "Graph Phase" <- w372
          }
          frame #1 {
            # "derivatives"
            # "frequencies"
            n204 = property on="Tab Control QControl" class="TabCtl (strict)"() -> ("Pages"=w404:refnum<vi>[])  [unwired: 2 in, 2 out]
            n205 = local read "Q Control En"() -> (w403:bool)
            n206 = Index Array(array=w404) -> (element #3=w406:refnum<vi>)  [unwired: 3 in, 2 out]
            n207 = property class="Page"(reference=w406, "PageEnb"=T4."Page Disabled & Grayed" ("Page Enabled State")) -> ()  [unwired: 1 in, 2 out]
            n208 = property on="Graph Phase" class="XYGraph (strict)"("DisabledEnum"=T5."Enabled" ("Disabled")) -> ()  [unwired: 2 in, 2 out]
            n209 = property on="Graph Amplitude" class="XYGraph (strict)"("DisabledEnum"=T5."Enabled" ("Disabled")) -> ()  [unwired: 2 in, 2 out]
            n210 = Boolean To (0,1)(Boolean=w403) -> (0, 1=w402:i16)
            n211 = Array Max & Min(array=w411) -> (min value=w426:dbl, min index (indices)=w430:i32)  [unwired: 2 out]
            n212 = Index Array(array=w412, index=w430) -> (element=w401:dbl)
            n213 = property on="Run Sweep" class="Bool (strict)"("DisabledEnum"=T5."Enabled" ("Disabled"), "Value"=FALSE ("Run")) -> ()  [unwired: 2 in, 2 out]
            n214 = Index Array(array=w410, index (row)=w402) -> (element=w413:refnum<vi>[])  [unwired: 1 in]
            n215 = for {
              tunnel: w413 -> [w441] mode=indexing
              n216 = Not A Number/Path/Refnum?(number/path/refnum=w441) -> (NaN/Path/Refnum?=w442:bool)
              n217 = case shown="False" w442 {
                tunnel: w441 -> [w445 _]
                tunnel: T5."Enabled" ("Disabled") -> [w444 _]
                frame #0 {
                  n218 = property class="DigNum (strict)"(reference=w445, "DisabledEnum"=w444) -> ()  [unwired: 1 in, 2 out]
                }
                frame #1 {
                }
              }
            }
            n219 = Divide(x=6.283185307179586, y=360.0 ("value")) -> (x/y=w427:dbl)
            n220 = Compound Arithmetic op=MULTIPLY(w427, w401, w426, -0.5 ("value")) -> (w416:dbl)
            n221 = disable-structure shown="Disabled" {
              disable-tunnel: [w436 "controlled" ("Cursor.Cursor Name")] -> w417
              disable-tunnel: w416 -> [w434 _]
              disable-tunnel: [w433 "native" ("Cursor.Cursor Name")] -> w415
              frame #0 {
                n222 = Format Into String(format string="controlled\nQ=%f" ("Cursor.Cursor Name"), w434) -> (resulting string=w436:string)  [unwired: 2 in, 1 out]
                n223 = Format Into String(format string="native\nQ=%f" ("Cursor.Cursor Name"), w434) -> (resulting string=w433:string)  [unwired: 2 in, 1 out]
              }
              frame #1 {
              }
            }
            n224 = Select(t=w417, s=w403, f=w415) -> (s? t:f=w424:string)
            n225 = for {
              tunnel: w414 -> [w454] mode=indexing
              tunnel: w402 -> [w446]
              tunnel: w401 -> [w453]
              tunnel: w424 -> [w452]
              tunnel: [w451] -> w423 mode=indexing
              n226 = property class="XYGraph (strict)"(reference=w454, "Active Cursor"=w446, "Cursor.Visible"=TRUE, "Cursor.Cursor X"=w453, "Cursor.Cursor Name"=w452, "Cursor.Cursor Name Visible"=TRUE ("Cursor Legend Visible"), "Cursor.Cursor Color"=u32 16771584, "Cursor.Cursor Style"=u8 1, "Cursor.Cursor Plot"=w446) -> ("Cursor.Cursor Y"=w451:dbl)  [unwired: 1 in, 2 out]
            }
            n227 = local read "AutoCenter"() -> (w409:bool)
            n228 = Multiply(x=2, y=w416) -> (x*y=w419:dbl)
            n229 = Index Array(array=w423) -> (element #1=w421:dbl, element #2=w422:dbl)  [unwired: 2 in]
            n230 = Divide(x=w401, y=w419) -> (x/y=w418:dbl)
            n231 = case shown="True" w409 {
              tunnel: w401 -> [_ w440]
              frame #0 {
              }
              frame #1 {
                n232 = property on="Center Frequency (Hz)" class="DigNum (strict)"("Val(Sgnl)"=w440) -> ()  [unwired: 2 in, 2 out]
              }
            }
            n233 = case shown="False" w403 {
              tunnel: w401 -> [w460 w463]
              tunnel: w416 -> [w461 w464]
              tunnel: w422 -> [w458 _]
              tunnel: w421 -> [w459 _]
              tunnel: w418 -> [w456 w462]
              frame #0 {
                w455 = T5."Enabled" ("Disabled")
                n234 = property on="Q Enhancement" class="Slide (strict)"() -> ("Value"=w457:dbl)  [unwired: 2 in, 2 out]
                n235 = property on="f/2Q (Hz)" class="DigNum (strict)"("Val(Sgnl)"=w456) -> ()  [unwired: 2 in, 2 out]
                n236 = property on="Resonance Freq (Hz)" class="DigNum (strict)"("Val(Sgnl)"=w460) -> ()  [unwired: 2 in, 2 out]
                n237 = property on="Q Enhancement" class="Slide (strict)"("Val(Sgnl)"=w457) -> ()  [unwired: 2 in, 2 out]
                n238 = property on="PID Drive Limit (V)" class="DigNum (strict)"("DisabledEnum"=w455) -> ()  [unwired: 2 in, 2 out]
                n239 = property on="Q Enhancement" class="Slide (strict)"("DisabledEnum"=w455) -> ()  [unwired: 2 in, 2 out]
                n240 = property on="Q Control En" class="Bool (strict)"("DisabledEnum"=w455) -> ()  [unwired: 2 in, 2 out]
                n241 = property on="Phase Shift (°)" class="DigNum (strict)"("Val(Sgnl)"=w458) -> ()  [unwired: 2 in, 2 out]
                "Q Factor" <- w461
                "Gain Margin (dB)" <- w459
              }
              frame #1 {
                n242 = property on="Characteristic Frequency Q" class="DigNum (strict)"("Val(Sgnl)"=w462) -> ()  [unwired: 2 in, 2 out]
                "controlled" <- w464
                "Resonance Frequency Q" <- w463
              }
            }
          }
        }
      }
    }
    n243 = local read "stop"() -> (w86:bool)
  }
  n244 = while {
    shift-right: [w469] -> w58
    shift-left: w59 -> [w470]
    shift-right: [w467] -> w56
    shift-left: w57 -> [w468]
    tunnel: w55 -> [w466]
    tunnel: w29 -> [w465]
    stop <- w472 stop-if-true
    n245 = event shown="[0] Timeout" {
      selector: _ -> [_ _ _ _ _ _ _ _ _ _ _ _ _ _ _ _ _ _ _ _]
      dyn-events: _ -> [_ _ _ _ _ _ _ _ _ _ _ _ _ _ _ _ _ _ _ _]
      timeout: 50 -> [_ _ _ _ _ _ _ _ _ _ _ _ _ _ _ _ _ _ _ _]
      tunnel: w470 -> [w474 w477 w487 w497 w515 w530 w560 w574 w590 w592 w599 w604 w608 w616 w620 w636 w640 w653 w676 w700]
      tunnel: [w474 w477 w484 w494 w522 w546 w560 w574 w590 w592 w599 w604 w608 w616 w620 w636 w640 w653 w675 w699] -> w469
      tunnel: w468 -> [w473 w476 w486 w496 w512 w527 w559 w573 w589 w591 w598 w603 w607 w615 w619 w635 w639 w652 w673 w697]
      tunnel: [w473 w476 w483 w493 w521 w545 w559 w573 w589 w591 w598 w603 w607 w615 w619 w635 w639 w652 w674 w698] -> w467
      tunnel: w466 -> [_ _ _ _ _ _ _ _ w587 w593 _ _ _ _ _ _ _ _ _ _]
      tunnel: w465 -> [_ _ _ _ _ _ _ _ _ _ _ _ _ _ w622 _ _ _ _ _]
      event #0 {
        n246 = event-data() -> ()  [unwired: 1 in, 2 out]
      }
      event #1 {
        n247 = event-data() -> ()  [unwired: 1 in, 2 out]
        n248 = local write "stop"(TRUE ("stop")) -> ()
      }
      event #2 {
        n249 = event-data() -> ("NewVal"=w485:dbl)  [unwired: 1 in, 4 out]
        n250 = local read "HW Channel"() -> (w479:i32)
        n251 = Equal To 0?(x=w479) -> (x = 0?=w478:bool)
        n252 = Select(t="demods/0/phaseshift" ("Path"), s=w478, f="demods/3/phaseshift") -> (s? t:f=w480:string)
        n253 = call-poly <instrlib>:"ziSetValue.vi"("Error In"=w486, "Value"=w485, "Path"=w480, "Handle In"=w487) -> ("Error Out"=w483:errorcluster, "Handle Out"=w484:T6)  [unwired: 1 in]
      }
      event #3 {
        n254 = event-data() -> ("NewVal"=w495:dbl)  [unwired: 1 in, 4 out]
        n255 = local read "PIDs"() -> (w488:i32)
        n256 = Index Array(array=dbl[][] [[0.0, 1.0], [2.0, 3.0]], index (row)=w488) -> (element=w490:dbl[])  [unwired: 1 in]
        n257 = for {
          tunnel: "pids/%u/range" ("Path") -> [w506]
          tunnel: w490 -> [w505] mode=indexing
          tunnel: [w504] -> w489 mode=indexing
          n258 = Format Into String(format string=w506, w505) -> (resulting string=w504:string)  [unwired: 2 in, 1 out]
        }
        n259 = for {
          tunnel: w495 -> [w501]
          shift-right: [w500] -> w494
          shift-left: w497 -> [w503]
          tunnel: w489 -> [w498] mode=indexing
          shift-right: [w499] -> w493
          shift-left: w496 -> [w502]
          n260 = call-poly <instrlib>:"ziSetValue.vi"("Error In"=w502, "Value"=w501, "Path"=w498, "Handle In"=w503) -> ("Error Out"=w499:errorcluster, "Handle Out"=w500:T6)  [unwired: 1 in]
        }
      }
      event #4 {
        n261 = event-data() -> ("NewVal"=w509:dbl)  [unwired: 1 in, 4 out]
        n262 = local read "Output Demod"() -> (w518:i32)
        n263 = local read "HW Channel"() -> (w517:i32)
        n264 = local read "HW Channel"() -> (w519:i32)
        n265 = Format Into String(format string="sigouts/%u/amplitudes/%u" ("Cursor.Cursor Name"), w517, w518) -> (resulting string=w507:string)  [unwired: 2 in, 1 out]
        n266 = Format Into String(format string="sigouts/%u/range" ("Cursor.Cursor Name"), w519) -> (resulting string=w511:string)  [unwired: 2 in, 1 out]
        n267 = call <instrlib>:"ziGetValueDouble.vi"("error in"=w512, "Path"=w511, "Handle in"=w515) -> ("error out"=w513:errorcluster, "Value"=w510:dbl, "Handle out"=w514:T6)
        n268 = Divide(x=w509, y=w510) -> (x/y=w508:dbl)
        n269 = call-poly <instrlib>:"ziSetValue.vi"("Error In"=w513, "Value"=w508, "Path"=w507, "Handle In"=w514) -> ("Error Out"=w521:errorcluster, "Handle Out"=w522:T6)  [unwired: 1 in]
      }
      event #5 {
        n270 = event-data() -> ()  [unwired: 1 in, 5 out]
        n271 = local read "Oscillator"() -> (w524:i32)
        n272 = local read "Center Frequency (Hz)"() -> (w526:dbl)
        n273 = Format Into String(format string="oscs/%u/freq", w524) -> (resulting string=w523:string)  [unwired: 2 in, 1 out]
        n274 = local read "HW Channel"() -> (w539:i32)
        n275 = local read "Bandwidth (Hz)"() -> (w540:dbl)
        n276 = call-poly <instrlib>:"ziSetValue.vi"("Error In"=w527, "Value"=w526, "Path"=w523, "Handle In"=w530) -> ("Error Out"=w528:errorcluster, "Handle Out"=w529:T6)  [unwired: 1 in]
        n277 = Equal To 0?(x=w539) -> (x = 0?=w535:bool)
        n278 = Select(t=string[] ["demods/0/timeconstant"], s=w535, f=string[] ["demods/4/timeconstant"]) -> (s? t:f=w536:string[])
        n279 = call <instrlib>:"ziBW2TC.vi"("Order (1)"=4 ("Order (#)"), "BW (Hz)"=w540) -> ("TC (s)"=w531:dbl)  [unwired: 1 in]
        n280 = for {
          shift-right: [w550] -> w543
          shift-left: w529 -> [w552]
          shift-right: [w549] -> w542
          shift-left: w528 -> [w551]
          tunnel: w531 -> [w548]
          tunnel: w536 -> [w547] mode=indexing
          n281 = call-poly <instrlib>:"ziSetValue.vi"("Error In"=w551, "Value"=w548, "Path"=w547, "Handle In"=w552) -> ("Error Out"=w549:errorcluster, "Handle Out"=w550:T6)  [unwired: 1 in]
        }
        n282 = Select(t=string[] ["demods/0/oscselect", "demods/1/oscselect", "demods/2/oscselect"], s=w535, f=string[] ["demods/3/oscselect", "demods/4/oscselect", "demods/5/oscselect"]) -> (s? t:f=w532:string[])
        n283 = for {
          shift-right: [w556] -> w546
          shift-left: w543 -> [w558]
          shift-right: [w555] -> w545
          shift-left: w542 -> [w557]
          tunnel: "Oscillator" -> [w554]
          tunnel: w532 -> [w553] mode=indexing
          n284 = call-poly <instrlib>:"ziSetValue.vi"("Error In"=w557, "Value"=w554, "Path"=w553, "Handle In"=w558) -> ("Error Out"=w555:errorcluster, "Handle Out"=w556:T6)  [unwired: 1 in]
        }
      }
      event #6 {
        n285 = event-data() -> ()  [unwired: 1 in, 5 out]
        n286 = disable-structure shown="Disabled" {
          frame #0 {
            n287 = local read "Characteristic Frequency Q"() -> (w566:dbl)
            n288 = local read "f/2Q (Hz)"() -> (w565:dbl)
            n289 = local read "Q Control En"() -> (w567:bool)
            n290 = Select(t=w566, s=w567, f=w565) -> (s? t:f=w564:dbl)
            n291 = Multiply(x=0.3, y=w564) -> (x*y=w563:dbl)
            n292 = local read "AutoBW"() -> (w561:bool)
            n293 = case shown="True" w561 {
              tunnel: [T5."Enabled" ("Disabled") T5."Disabled and Grayed Out" ("Disabled")] -> w568
              tunnel: w563 -> [_ w570]
              frame #0 {
              }
              frame #1 {
                n294 = local write "BW (Hz)"(w570) -> ()
              }
            }
            n295 = property on="BW (Hz)" class="DigNum (strict)"("DisabledEnum"=w568) -> ()  [unwired: 2 in, 2 out]
          }
          frame #1 {
          }
        }
      }
      event #7 {
        n296 = event-data() -> ("NewVal"=w578:dbl)  [unwired: 1 in, 4 out]
        n297 = local read "Gain Margin (dB)"() -> (w582:dbl)
        n298 = Less?(x=w578, y=1.0) -> ()  [unwired: 1 out]
        n299 = Reciprocal(x=w578) -> (1/x=w579:dbl)
        n300 = expression code="10**(x/20)"(w582) -> (w581:dbl)
        n301 = Subtract(x=1.0, y=w579) -> (x-y=w580:dbl)
        n302 = Divide(x=w580, y=w581) -> (x/y=w576:dbl)
        n303 = case shown="False" TRUE {
          tunnel: w576 -> [w585 w586]
          tunnel: [w584 w586] -> w575
          frame #0 {
            n304 = Negate(x=w585) -> (-x=w584:dbl)
          }
          frame #1 {
          }
        }
        n305 = property on="Feedback Gain (V/Vrms)" class="Slide (strict)"("Val(Sgnl)"=w575) -> ()  [unwired: 2 in, 2 out]
      }
      event #8 {
        n306 = event-data() -> ()  [unwired: 1 in, 5 out]
        n307 = Enqueue Element(queue=w587, element="setup" ("notification")) -> ()  [unwired: 2 in, 3 out]
      }
      event #9 {
        n308 = event-data() -> ()  [unwired: 1 in, 5 out]
        n309 = Enqueue Element(queue=w593, element="sweep" ("notification")) -> ()  [unwired: 2 in, 3 out]
      }
      event #10 {
        n310 = event-data() -> ("NewVal"=w596:dbl)  [unwired: 1 in, 4 out]
        n311 = local read "AutoCenter"() -> (w595:bool)
        n312 = case shown="True" w595 {
          tunnel: w596 -> [_ w600]
          frame #0 {
          }
          frame #1 {
            n313 = local write "Center Frequency (Hz)"(w600) -> ()
          }
        }
        n314 = property on="AutoCenter" class="Bool (strict)"("DisabledEnum"=T5."Enabled" ("Disabled")) -> ()  [unwired: 2 in, 2 out]
      }
      event #11 {
        n315 = event-data() -> ("NewVal"=w602:dbl)  [unwired: 1 in, 4 out]
        n316 = local read "AutoPhase"() -> (w601:bool)
        n317 = case shown="True" w601 {
          tunnel: w602 -> [_ w606]
          frame #0 {
          }
          frame #1 {
            n318 = Negate(x=w606) -> (-x=w605:dbl)
            n319 = property on="Feedback Phase (deg)" class="Slide (strict)"("Val(Sgnl)"=w605) -> ()  [unwired: 2 in, 2 out]
          }
        }
      }
      event #12 {
        n320 = event-data() -> ("NewVal"=w609:bool)  [unwired: 1 in, 4 out]
        n321 = case shown="True" w609 {
          frame #0 {
          }
          frame #1 {
            n322 = local read "Resonance Freq (Hz)"() -> (w610:dbl)
            n323 = local write "Center Frequency (Hz)"(w610) -> ()
          }
        }
      }
      event #13 {
        n324 = event-data() -> ("NewVal"=w611:bool)  [unwired: 1 in, 4 out]
        n325 = case shown="True" w611 {
          frame #0 {
          }
          frame #1 {
            n326 = local read "Phase Shift (°)"() -> (w617:dbl)
            n327 = Negate(x=w617) -> (-x=w618:dbl)
            n328 = property on="Feedback Phase (deg)" class="Slide (strict)"("Val(Sgnl)"=w618) -> ()  [unwired: 2 in, 2 out]
          }
        }
        n329 = Select(t=T5."Disabled and Grayed Out" ("Disabled"), s=w611, f=T5."Enabled" ("Disabled")) -> (s? t:f=w614:T5)
        n330 = property on="Feedback Phase (deg)" class="Slide (strict)"("DisabledEnum"=w614) -> ()  [unwired: 2 in, 2 out]
      }
      event #14 {
        n331 = event-data() -> ("NewVal"=w621:bool)  [unwired: 1 in, 4 out]
        n332 = for {
          tunnel: w622 -> [w626] mode=indexing
          tunnel: w621 -> [w624]
          n333 = property class="XYGraph (strict)"(reference=w626, "Active Plot"=u32 2, "Plot.Visible?"=w624) -> (error out=w623:errorcluster)  [unwired: 1 in, 1 out]
          n334 = call <vilib>:"Clear Errors.vi"("error in (no error)"=w623) -> ()  [unwired: 6 in, 1 out]
        }
      }
      event #15 {
        n335 = event-data() -> ("NewVal"=w629:bool)  [unwired: 1 in, 4 out]
        n336 = control-ref of="ADC Over"() -> (w627:refnum<vi>)
        n337 = control-ref of="Stability Warning"() -> (w628:refnum<vi>)
        n338 = control-ref of="Feedback Gain (V/Vrms)"() -> (w634:refnum<vi>)
        n339 = Build Array(w627, w628, w634) -> (w633:refnum<vi>[])
        n340 = Select(t=T5."Disabled and Grayed Out" ("Disabled"), s=w629, f=T5."Enabled" ("Disabled")) -> (s? t:f=w632:T5)
        n341 = for {
          tunnel: w633 -> [w638] mode=indexing
          tunnel: w632 -> [w637]
          n342 = property class="Ctl"(reference=w638, "DisabledEnum"=w637) -> ()  [unwired: 1 in, 2 out]
        }
      }
      event #16 {
        n343 = event-data() -> ("CtlRef"=w644:refnum<vi>, "NewVal"=w643:dbl)  [unwired: 1 in, 3 out]
        n344 = local read "BW (Hz)"() -> (w642:dbl)
        n345 = Less?(x=w643, y=w642) -> (x < y?=w641:bool)
        n346 = property class="DigNum (strict)"(reference=w644, "Blinking"=w641) -> ()  [unwired: 1 in, 2 out]
      }
      event #17 {
        n347 = event-data() -> ("CtlRef"=w654:refnum<vi>, "NewVal"=w649:dbl)  [unwired: 1 in, 3 out]
        n348 = control-ref of="f/2Q (Hz)"() -> (w648:refnum<vi>)
        n349 = control-ref of="Characteristic Frequency Q"() -> (w647:refnum<vi>)
        n350 = Build Array(w648, w647) -> (w645:refnum<vi>[])
        n351 = for {
          shift-right: [w665] -> w650
          shift-left: FALSE ("x > y?") -> [w664]
          tunnel: w649 -> [w662]
          tunnel: [w660] -> w646 mode=indexing
          tunnel: w645 -> [w657] mode=indexing
          n352 = property class="DigNum (strict)"(reference=w657) -> ("DisabledEnum"=w659:T5, "Value"=w658:dbl)  [unwired: 1 in, 2 out]
          n353 = Less?(x=w658, y=w662) -> (x < y?=w661:bool)
          n354 = Equal?(x=T5."Enabled" ("DisabledEnum"), y=w659) -> (x = y?=w663:bool)
          n355 = And(x=w663, y=w661) -> (x .and. y?=w660:bool)
          n356 = Or(x=w660, y=w664) -> (x .or. y?=w665:bool)
        }
        n357 = property class="DigNum (strict)"(reference=w654, "Blinking"=w650) -> ()  [unwired: 1 in, 2 out]
        n358 = for {
          tunnel: w646 -> [w656] mode=indexing
          tunnel: w645 -> [w655] mode=indexing
          n359 = property class="DigNum (strict)"(reference=w655, "Blinking"=w656) -> ()  [unwired: 1 in, 2 out]
        }
      }
      event #18 {
        n360 = event-data() -> ("NewVal"=w667:bool)  [unwired: 1 in, 4 out]
        n361 = local read "HW Channel"() -> (w668:i32)
        n362 = Equal To 0?(x=w668) -> (x = 0?=w669:bool)
        n363 = Boolean To (0,1)(Boolean=w667) -> (0, 1=w677:i16)
        n364 = Select(t=string[] ["sigouts/0/enables/1", "sigouts/0/enables/2"], s=w669, f=string[] ["sigouts/1/enables/4", "sigouts/1/enables/5"]) -> (s? t:f=w672:string[])
        n365 = for {
          tunnel: w677 -> [w683]
          tunnel: w672 -> [w682] mode=indexing
          shift-right: [w680] -> w675
          shift-left: w676 -> [w681]
          shift-right: [w679] -> w674
          shift-left: w673 -> [w678]
          n366 = call-poly <instrlib>:"ziSetValue.vi"("Error In"=w678, "Value"=w683, "Path"=w682, "Handle In"=w681) -> ("Error Out"=w679:errorcluster, "Handle Out"=w680:T6)  [unwired: 1 in]
        }
      }
      event #19 {
        n367 = event-data() -> ("NewVal"=w684:dbl)  [unwired: 1 in, 4 out]
        n368 = local read "Gain Margin (dB)"() -> (w695:dbl)
        n369 = local read "PIDs"() -> (w686:i32)
        n370 = Index Array(array=dbl[][] [[0.0, 1.0], [2.0, 3.0]], index (row)=w686) -> (element=w687:dbl[])  [unwired: 1 in]
        n371 = for {
          tunnel: "pids/%u/P" -> [w707]
          tunnel: w687 -> [w706] mode=indexing
          tunnel: [w705] -> w685 mode=indexing
          n372 = Format Into String(format string=w707, w706) -> (resulting string=w705:string)  [unwired: 2 in, 1 out]
        }
        n373 = expression code="10**(x/20)"(w695) -> (w694:dbl)
        n374 = Multiply(x=w694, y=w684) -> (x*y=w693:dbl)
        n375 = Subtract(x=1.0, y=w693) -> (x-y=w692:dbl)
        n376 = for {
          tunnel: w700 -> [w713]
          tunnel: [w712] -> w699
          tunnel: [w711] -> w698
          tunnel: w697 -> [w710]
          tunnel: w684 -> [w709]
          tunnel: w685 -> [w708] mode=indexing
          n377 = call-poly <instrlib>:"ziSetValue.vi"("Error In"=w710, "Value"=w709, "Path"=w708, "Handle In"=w713) -> ("Error Out"=w711:errorcluster, "Handle Out"=w712:T6)  [unwired: 1 in]
        }
        n378 = Reciprocal(x=w692) -> (1/x=w690:dbl)
        n379 = Less Than 0?(x=w692) -> (x < 0?=w691:bool)
        "Stability Warning" <- w691
        n380 = disable-structure shown="Disabled" {
          disable-tunnel: w691 -> [w704 _]
          disable-tunnel: w690 -> [w702 _]
          frame #0 {
            n381 = Select(t=inf, s=w704, f=w702) -> (s? t:f=w703:dbl)
            n382 = property on="Q Enhancement" class="Slide (strict)"("Value"=w703) -> ()  [unwired: 2 in, 2 out]
          }
          frame #1 {
          }
        }
      }
    }
    n383 = local read "stop"() -> (w472:bool)
  }
  n384 = while {
    shift-right: [w726] -> w54
    shift-left: w25 -> [w728]
    shift-right: [w725] -> w53
    shift-left: w24 -> [w727]
    stop <- w729 stop-if-true
    n385 = call <instrlib>:"ziPollDataEx.vi"("error in"=w727, "Timeout ms (50)"=50 ("TimeOut ms (50)"), "Handle In"=w728) -> ("error out"=w725:errorcluster, "PathArray"=w722:string[], "Handle Out"=w726:T6, "Value Double"=w716:dbl, "Timed Out"=w714:bool, "Value Int"=w715:i32)  [unwired: 1 in, 2 out]
    n386 = Index Array(array=w722, index #1=1 ("index")) -> (element #1=w718:string, element #2=w717:string)  [unwired: 1 in]
    n387 = local read "HW Channel"() -> (w721:i32)
    n388 = Decimal String To Number(string=w717) -> (number=w720:i32)  [unwired: 2 in, 1 out]
    n389 = Equal?(x=w720, y=w721) -> (x = y?=w719:bool)
    n390 = case shown="True" w714 {
      tunnel: w716 -> [w733 _]
      tunnel: w719 -> [w732 _]
      tunnel: w718 -> [w731 _]
      tunnel: w715 -> [w730 _]
      frame #0 {
        n391 = case shown="Default" w731 {
          tunnel: w733 -> [_ _ w737]
          tunnel: w732 -> [_ _ w736]
          tunnel: w730 -> [w734 _ _]
          frame #0 {
            n392 = Not Equal To 0?(x=w734) -> (x != 0?=→"ADC Over":bool)
          }
          frame #1 {
          }
          frame #2 {
            n393 = case shown="False" w736 {
              tunnel: w737 -> [_ w738]
              frame #0 {
              }
              frame #1 {
                w745 = 1.0 ("upper limit")
                n394 = local read "fmax"() -> (w740:dbl)
                n395 = local read "fmin"() -> (w739:dbl)
                n396 = Subtract(x=w738, y=w739) -> (x-y=w747:dbl)
                n397 = Subtract(x=w740, y=w739) -> (x-y=w748:dbl)
                n398 = Divide(x=w747, y=w748) -> (x/y=w744:dbl)
                n399 = Equal?(x=w744, y=w745) -> (x = y?=w741:bool)
                n400 = In Range and Coerce(upper limit=w745, x=w744, lower limit=0.0) -> (In Range?=w742:bool)  [unwired: 1 out]
                n401 = Or(x=w741, y=w742) -> (x .or. y?=w743:bool)
                n402 = case shown="True" w743 {
                  tunnel: w744 -> [_ w749]
                  frame #0 {
                  }
                  frame #1 {
                    n403 = local write "Sweep Progress"(w749) -> ()
                  }
                }
              }
            }
          }
        }
      }
      frame #1 {
      }
    }
    n404 = local read "stop"() -> (w729:bool)
  }
  n405 = call <instrlib>:"ziClose.vi"("Error In"=w56, "Handle In"=w58) -> ("Error Out"=w22:errorcluster)  [unwired: 2 in, 1 out]
  n406 = call <instrlib>:"ziClose.vi"("Error In"=w53, "Handle In"=w54) -> ("Error Out"=w21:errorcluster)  [unwired: 2 in, 1 out]
  n407 = case shown="False" "restore settings" {
    tunnel: w35 -> [_ w756]
    tunnel: w34 -> [w751 w755]
    tunnel: w33 -> [w750 w754]
    tunnel: [w751 w753] -> w32
    tunnel: [w750 w752] -> w31
    frame #0 {
    }
    frame #1 {
      n408 = call <instrlib>:"ziLoadSettings.vi"("Error in"=w754, "File path (dialog if empty)"=w756, "Handle in"=w755) -> ("Error out"=w752:errorcluster, "Handle out"=w753:T6)  [unwired: 2 in]
    }
  }
  n409 = call <instrlib>:"ziClose.vi"("Error In"=w31, "Handle In"=w32) -> ("Error Out"=w23:errorcluster)  [unwired: 2 in, 1 out]
  n410 = flat-sequence "Quit if running in compiled form" {
    tunnel: w23 -> [_]
    tunnel: w22 -> [_]
    tunnel: w21 -> [_]
    frame #0 {
      n411 = property class="App"() -> ("App.Kind"=w760:T10)  [unwired: 2 in, 2 out]
      n412 = local write "stop"(FALSE ("stop")) -> ()
      n413 = Equal?(x=w760, y=T10."Run Time System" ("Application:Kind")) -> (x = y?=w758:bool)
      n414 = Quit LabVIEW(quit? (T)=w758) -> ()
    }
  }
